vi "BIAS_Client_2.vi"() -> ()   [LabVIEW 2012]
uses:
  <userlib>/BIAS2/subvis/ROI_rect.ctl
  <userlib>/BIAS2/subvis/Imaging_State.ctl
  <userlib>/BIAS2/subvis/Frame_Controls.ctl
  <userlib>/BIAS2/subvis/ui/CameraParameters.ctl
  <vilib>/Utility/error.llb/DialogType.ctl
  <userlib>/BIAS2/subvis/zlock/ZLock.lvclass
  <userlib>/BIAS2/classes/CameraBase/CameraBase.lvclass
  <userlib>/BIAS2/subvis/ExposureSettings.ctl
  <vilib>/addons/h5labview2/file/H5Fmode.ctl
  <vilib>/event_ctls.llb/lveventtype.ctl
  <vilib>/addons/h5labview2/base/lib_path.vi
  <vilib>/addons/h5labview2/base/H5Equery.vi
  <vilib>/Utility/file.llb/Read From Spreadsheet File (DBL).vi
  <vilib>/addons/h5labview2/attrib/H5Aread.llb/H5Aread.xnode
  <vilib>/addons/h5labview2/dataset/H5Dread.llb/H5Dread.xnode
  <vilib>/addons/h5labview2/attrib/H5Awrite.llb/H5Awrite.xnode
  <vilib>/Analysis/NI_AALPro.lvlib
  <vilib>/addons/h5labview2/file/H5F.lvlib
  <vilib>/addons/h5labview2/group/H5G.lvlib
  <vilib>/addons/h5labview2/attrib/H5A.lvlib
panel:
  in  "files":T1 caption="Files"
  in  "stop":bool
  in  "tools_zoom":T2 caption="Zoom tools"
  in  "tools_view":cluster{"sel":bool, "in":bool, "out":bool} caption="View tools"
  in  "capture":T3 caption="Capture"
  out "stop_time":dbl=11.582550000000003
  out "busy":bool caption="Busy"
  out "recent_error":bool caption="Error"
  out "remote":bool caption="Remote"
  out "acquiring":bool caption="Acquiring"
  out "img_OD":T4(plugin-control)
  out "image_raw":sgl[][](array[numeric])
  in  "tabs":T5(tab)
  in  "binning":cluster{"x":u8, "y":u8}={"x"=1, "y"=1}
  in  "effective_pixel":dbl=5.9e-06 caption="effective pixel size"
  in  "rotation":u16(ring) items=["Do not rotate", "Rotate 90°", "Rotate 180°", "Rotate -90°"]
  out "cam_params":cluster{"String":string, "value":variant}[](array[cluster])=[{"String"="StatusInformation::LostBufferCount", "value"=variant(i64 0)}, {"String"="StatusInformation::LastBufferNumber", "value"=variant(u32 0)}, {"String"="StatusInformation::LastBufferCount", "value"=variant(i64 1)}, {"String"="StatusInformation::AcqInProgress", "value"=variant(bool FALSE)}, {"String"="CameraInformation::VendorName", "value"=variant(string "Point Grey Research")}, {"String"="CameraInformation::SerialNumberLow", "value"=variant(u32 11272219)}, {"String"="CameraInformation::SerialNumberHigh", "value"=variant(u32 11574529)}, {"String"="CameraInformation::ModelName", "value"=variant(string "Flea3 FL3-FW-03S1M")}, {"String"="CameraInformation::BusType", "value"=variant(string "FireWire")}, {"String"="CameraInformation::BaseAddress", "value"=variant(u32 4042260480)}, {"String"="CameraAttributes::TriggerDelay::Value", "value"=variant(dbl 0.0)}, {"String"="CameraAttributes::TriggerDelay::Mode", "value"=variant(string "Off")}, {"String"="CameraAttributes::Trigger::TriggerSource", "value"=variant(string "Source 0")}, {"String"="CameraAttributes::Trigger::TriggerParameter", "value"=variant(u32 0)}, {"String"="CameraAttributes::Trigger::TriggerMode", "value"=variant(string "Mode 1")}, {"String"="CameraAttributes::Trigger::TriggerActivation", "value"=variant(string "Level Low")}, {"String"="CameraAttributes::Trigger::SoftwareTrigger", "value"=variant(string "")}, {"String"="CameraAttributes::Temperature::Target", "value"=variant(dbl 2931.0)}, {"String"="CameraAttributes::Temperature::Mode", "value"=variant(string "UnknownEnumValue")}, {"String"="CameraAttributes::Temperature::Current", "value"=variant(dbl 3069.0)}, {"String"="CameraAttributes::Shutter::Value", "value"=variant(dbl 0.009999999776482582)}, {"String"="CameraAttributes::Shutter::Mode", "value"=variant(string "Absolute")}, {"String"="CameraAttributes::Sharpness::Value", "value"=variant(dbl 968.0)}, {"String"="CameraAttributes::Sharpness::Mode", "value"=variant(string "Off")}, {"String"="CameraAttributes::Gamma::Value", "value"=variant(dbl 1280.0)}, {"String"="CameraAttributes::Gamma::Mode", "value"=variant(string "Off")}, {"String"="CameraAttributes::Gain::Value", "value"=variant(dbl 10.0)}, {"String"="CameraAttributes::Gain::Mode", "value"=variant(string "Absolute")}, {"String"="CameraAttributes::FrameRate::Value", "value"=variant(dbl 480.0)}, {"String"="CameraAttributes::FrameRate::Mode", "value"=variant(string "Auto")}, {"String"="CameraAttributes::Brightness::Value", "value"=variant(dbl 0.0)}, {"String"="CameraAttributes::Brightness::Mode", "value"=variant(string "Absolute")}, {"String"="CameraAttributes::AutoExposure::Value", "value"=variant(dbl 6.0)}, {"String"="CameraAttributes::AutoExposure::Mode", "value"=variant(string "Off")}, {"String"="AcquisitionAttributes::Width", "value"=variant(u32 648)}, {"String"="AcquisitionAttributes::VideoMode", "value"=variant(string "Format 7, Mode 0, 648 x 488")}, {"String"="AcquisitionAttributes::Timeout", "value"=variant(u32 2000)}, {"String"="AcquisitionAttributes::SwapPixelBytes", "value"=variant(bool FALSE)}, {"String"="AcquisitionAttributes::Speed", "value"=variant(string "400 Mbps")}, {"String"="AcquisitionAttributes::ShiftPixelBits", "value"=variant(bool TRUE)}, {"String"="AcquisitionAttributes::ReserveDualPackets", "value"=variant(bool TRUE)}, {"String"="AcquisitionAttributes::ReceiveTimestampMode", "value"=variant(string "None")}, {"String"="AcquisitionAttributes::PixelSignedness", "value"=variant(string "Unsigned")}, {"String"="AcquisitionAttributes::PixelFormat", "value"=variant(string "Mono 16")}, {"String"="AcquisitionAttributes::PayloadSize", "value"=variant(u32 614400)}, {"String"="AcquisitionAttributes::PacketSize", "value"=variant(u32 3948)}, {"String"="AcquisitionAttributes::OverwriteMode", "value"=variant(string "Get Newest")}, {"String"="AcquisitionAttributes::OutputImageType", "value"=variant(string "Auto")}, {"String"="AcquisitionAttributes::OffsetY", "value"=variant(u32 0)}, {"String"="AcquisitionAttributes::OffsetX", "value"=variant(u32 0)}, {"String"="AcquisitionAttributes::IgnoreFirstFrame", "value"=variant(bool FALSE)}, {"String"="AcquisitionAttributes::Height", "value"=variant(u32 488)}, {"String"="AcquisitionAttributes::FrameInterval", "value"=variant(u32 19)}, {"String"="AcquisitionAttributes::Controller::StreamChannelMode", "value"=variant(string "Automatic")}, {"String"="AcquisitionAttributes::Controller::DesiredStreamChannel", "value"=variant(u32 0)}, {"String"="AcquisitionAttributes::BitsPerPixel", "value"=variant(string "12-bit")}, {"String"="AcquisitionAttributes::Bayer::Pattern", "value"=variant(string "Use hardware value")}, {"String"="AcquisitionAttributes::Bayer::GainR", "value"=variant(dbl 1.0)}, {"String"="AcquisitionAttributes::Bayer::GainG", "value"=variant(dbl 1.0)}, {"String"="AcquisitionAttributes::Bayer::GainB", "value"=variant(dbl 1.0)}, {"String"="AcquisitionAttributes::Bayer::Algorithm", "value"=variant(string "Bilinear")}] caption="Camera Parameters"
  in  "rois":T7(array[cluster])=[{"get"=FALSE, "set"=FALSE, "rect"={"left"=0, "top"=0, "right"=0, "bottom"=0}, "color"=16777224}, {"get"=FALSE, "set"=FALSE, "rect"={"left"=0, "top"=0, "right"=0, "bottom"=0}, "color"=6618880}, {"get"=FALSE, "set"=FALSE, "rect"={"left"=0, "top"=0, "right"=0, "bottom"=0}, "color"=16776960}, {"get"=FALSE, "set"=FALSE, "rect"={"left"=0, "top"=0, "right"=0, "bottom"=0}, "color"=4849919}]
  in  "camera name":string="XY_1_Flea3"
  out "camera model":string="Flea3 FL3-FW-03S1M, serial 0xB09D0100AC001B"
  in  "exposure":sgl=100.0 caption="exposure (ms)"
  out "location":string caption="camera location"
  out "roi_sensor":T6={"left"=0, "top"=0, "right"=640, "bottom"=480} caption="camera size"
  out "roi_capture":T6={"left"=0, "top"=0, "right"=640, "bottom"=480}
  out "keep":u8
  out "working dir":path
  out "current file":string
  in  "raw_ctrls":T8={"col_scheme"=0, "val_min"=100.0, "val_max"=16384.0, "automax"=FALSE} {"col_scheme" items=["Grayscale", "Rainbow", "Temperature", "-", "AlpineColors", "Amherst", "Aquamarine", "ArmyColors", "AtlanticColors", "AuroraColors", "AvocadoColors", "BeachColors", "BlueGreenYellow", "BrassTones", "BrightBands", "BrownCyanTones", "CandyColors", "CherryTones", "CMYKColors", "CoffeeTones", "DarkBands", "DarkRainbow", "DarkTerrain", "DeepSeaColors", "Default", "FallColors", "FruitPunchColors", "FuchsiaTones", "GrayTones", "GrayYellowTones", "GreenBrownTerrain", "GreenPinkTones", "IslandColors", "LabVIEW", "LakeColors", "LightTemperatureMap", "LightTerrain", "MintColors", "NeonColors", "NIST", "Pastel", "PearlColors", "PigeonTones", "PlumColors", "Rainbow", "RedBlueTones", "RedGreenSplit", "RoseColors", "RustTones", "SandyTerrain", "SiennaTones", "SolarColors", "SouthwestColors", "StarryNightColors", "SunsetColors", "TemperatureMap", "ThermometerColors", "ValentineTones", "WatermelonColors"]; "val_max" format="%_4g"; "val_min" format="%_4g"}
  in  "raw_list":i32(listbox)=-1 caption="Raw Frames"
  in  "hold_frames":bool caption="Hold last flat/dark frames"
  in  "histograms":bool caption="histogram"
  out "recent":string[](array[string])=["[31/10/14-12:50:53] Instance started, XY_1_Flea3"] caption="recent log messages"
  out "state":T9=enum."Quit" caption="system state"
  in  "last error":T10={"status"=FALSE, "code"=42, "description"="", "time"=timestamp(3029490000.67111 s since 1904-01-01)} caption="most recent error:" {"time" format="%<%H:%M:%S %d/%m/%y>T"}
  out "sequencer":T11(array[cluster])
  out "roi_current":T6
  out "image_data":u16[][][](array[numeric])
  out "frame":i32=-1 caption="display_frame"
  out "BLACS port":u16=1024
  out "image_size":i32[](array[numeric])
  out "attribs":variant[](array[variant])=[variant(i32 864), variant(i32 519), variant(i32 1176), variant(i32 878), variant(i64 0), variant(string "Freerun"), variant(u32 1), variant(u32 1), variant(i64 864), variant(i64 519), variant(i64 312), variant(i64 359), variant(dbl 100000.00149011612)]
  in  "Parameters":T12={"name"="XY_1_Flea3", "sdk"="IMAQdx_Flea3_Firewire", "serial"=49712223532875803, "port"=1024, "h5"=path "Y:/Experiments/rb_chip/connectiontable.h5", "zlock server"="localhost", "zlock port"=7339} {"serial" format="%x"}
  out "raw histograms":T13(array[cluster])
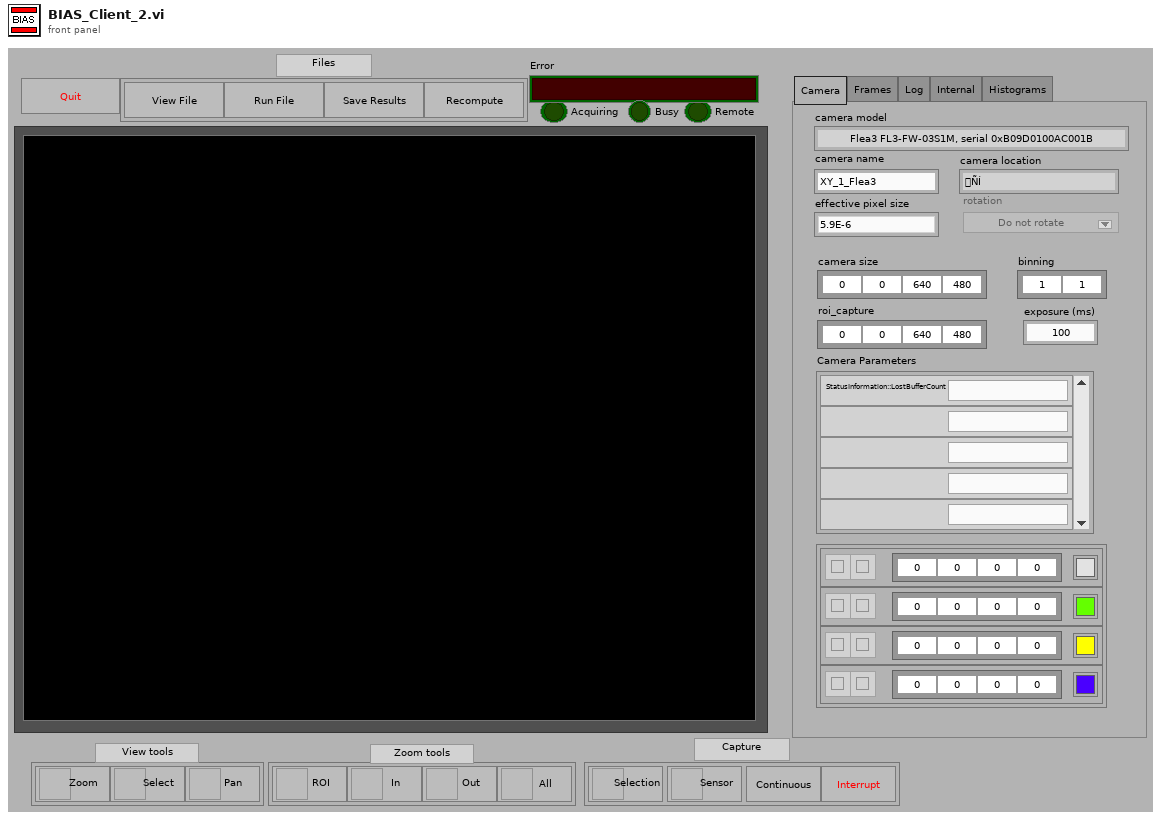
[diagram p1: front panel]
types:
  T1 = cluster{"open_file 2":bool, "open_file":bool, "save_file":bool, "open_file 3":bool}
  T2 = cluster{"sel":bool, "in":bool, "out":bool, "all":bool}
  T3 = cluster{"roi":bool, "chip":bool, "continuous":bool, "abort":bool}
  T4 = typedef "IMAQ Image.ctl" = refnum<image>
  T5 = enum32{"Camera", "Frames", "Log", "Internal", "Histograms"}
  T6 = typedef "ROI_rect.ctl" = cluster{"left":i32, "top":i32, "right":i32, "bottom":i32}
  T7 = cluster{"get":bool, "set":bool, "rect":T6, "color":u32}[]
  T8 = typedef "Frame_Controls.ctl" = cluster{"col_scheme":u16, "val_min":sgl, "val_max":sgl, "automax":bool}
  T9 = typedef "Imaging_State.ctl" = enum16{"<NULL>", "Init", "Read File", "Save File", "Idle", "Compute", "Redraw", "Draw Overlays", "Software trigger", "Acquire", "Fit", "Clear", "Quit"}
  T10 = cluster{"status":bool, "code":i32, "description":string, "time":timestamp}
  T11 = cluster{"name":string, "shots":string[], "ids":i32[]}[]
  T12 = typedef "CameraParameters.ctl" = cluster{"name":string, "sdk":string, "serial":u64, "port":u16, "h5":path, "zlock server":string, "zlock port":u32}
  T13 = cluster{"XY Graph":cluster{"X Values":dbl[], "Histogram: h(x)":i32[]}}[]
  T14 = typedef "DialogType.ctl" = u16
  T15 = typedef "ExposureSettings.ctl" = cluster{"exposure":dbl, "external":bool, "roi":T6, "frames":i32, "binning":cluster{"x":u8, "y":u8}}
  T16 = typedef "H5F.lvlib/H5Fmode.ctl" = enum16{"read-only", "read-write", "overwrite", "create new", "open or create"}
  T17 = typedef "Image Type" = u32
  T18 = cluster{"sensor_width":u16, "sensor_width":u16, "sensor_width":u16, "sensor_height":u16}
  T19 = cluster{"X Values":dbl[], "Histogram: h(x)":i32[]}
  T20 = cluster{"Histogram Graph":cluster{"X Values":dbl[], "Histogram: h(x)":i32[]}}
  T21 = typedef "hid_t.ctl" = i32
  T22 = cluster{"name":string, "shots":string[], i32[]}[]
  T23 = typedef "lveventtype.ctl" = enum32{"Null", "Timeout", "Annotation Menu Selection", "Annotation Menu Selection?", "App Instance Close", "App Instance Close?", "Autoscale Range Change", "Cell Edit", "Cell Edit?", "Cursor Grab", "Cursor Grab?", "Cursor Menu Selection", "Cursor Menu Selection?", "Cursor Move", "Cursor Release", "Data Change", "Direction Change", "Display State Change", "Drag Ended", "Drag Enter", "Drag Leave", "Drag Over", "Drag Source Update", "Drag Starting", "Drag Starting?", "Drop", "Exec State Change", "Key Down", "Key Down?", "Key Repeat", "Key Repeat?", "Key Up", "Listbox Double Click", "Menu Activation?", "Menu Selection (App)", "Menu Selection? (App)", "Menu Selection (User)", "Mouse Down", "Mouse Down?", "Mouse Enter", "Mouse Leave", "Mouse Move", "Mouse Up", "NI Security User Change (App)", "Pane Size", "Panel Close", "Panel Close?", "Panel Resize", "Plot Attribute Change", "Scale Range Change", "Shortcut Menu Activation?", "Shortcut Menu Selection (App)", "Shortcut Menu Selection? (App)", "Shortcut Menu Selection (User)", "Tree Double Click", "Tree Drag", "Tree Drag?", "Tree Drop", "Tree Drop?", "Tree Item Close", "Tree Item Close?", "Tree Item Open", "Tree Item Open?", "Value Change"}
  T24 = cluster{"Global Rectangle":i32[], "Contours":cluster{"Contour Type":u32, "ROI Type":u32, "Points":i32[]}[]}
  T25 = typedef "ROI Descriptor" = cluster{"Global Rectangle":i32[], "Contours":cluster{"ID":enum32{"External", "Internal"}, "Type":u32, "Coordinates":i32[]}[]}
  T26 = cluster{"Contour Type":u32, "ROI Type":u32, "Points":i32[]}[]
  T27 = cluster{"FinalVal[0]":bool, "FinalVal[1]":bool, "FinalVal[2]":bool}
  T28 = cluster{"all rows[0]":dbl, "all rows[1]":dbl, "all rows[2]":dbl}
  T29 = cluster{"get":bool, "set":bool, "rect":T6, "color":u32}
  T30 = cluster{"Value":u8, "Value":u8, "Value":u8, "Value":u8}
  T31 = cluster{"col_scheme":u16, "val_min":sgl, "val_max":sgl, "automax":bool}
  T32 = enum16{"Standard", "Buffered", "CRLF", "Immediate"}
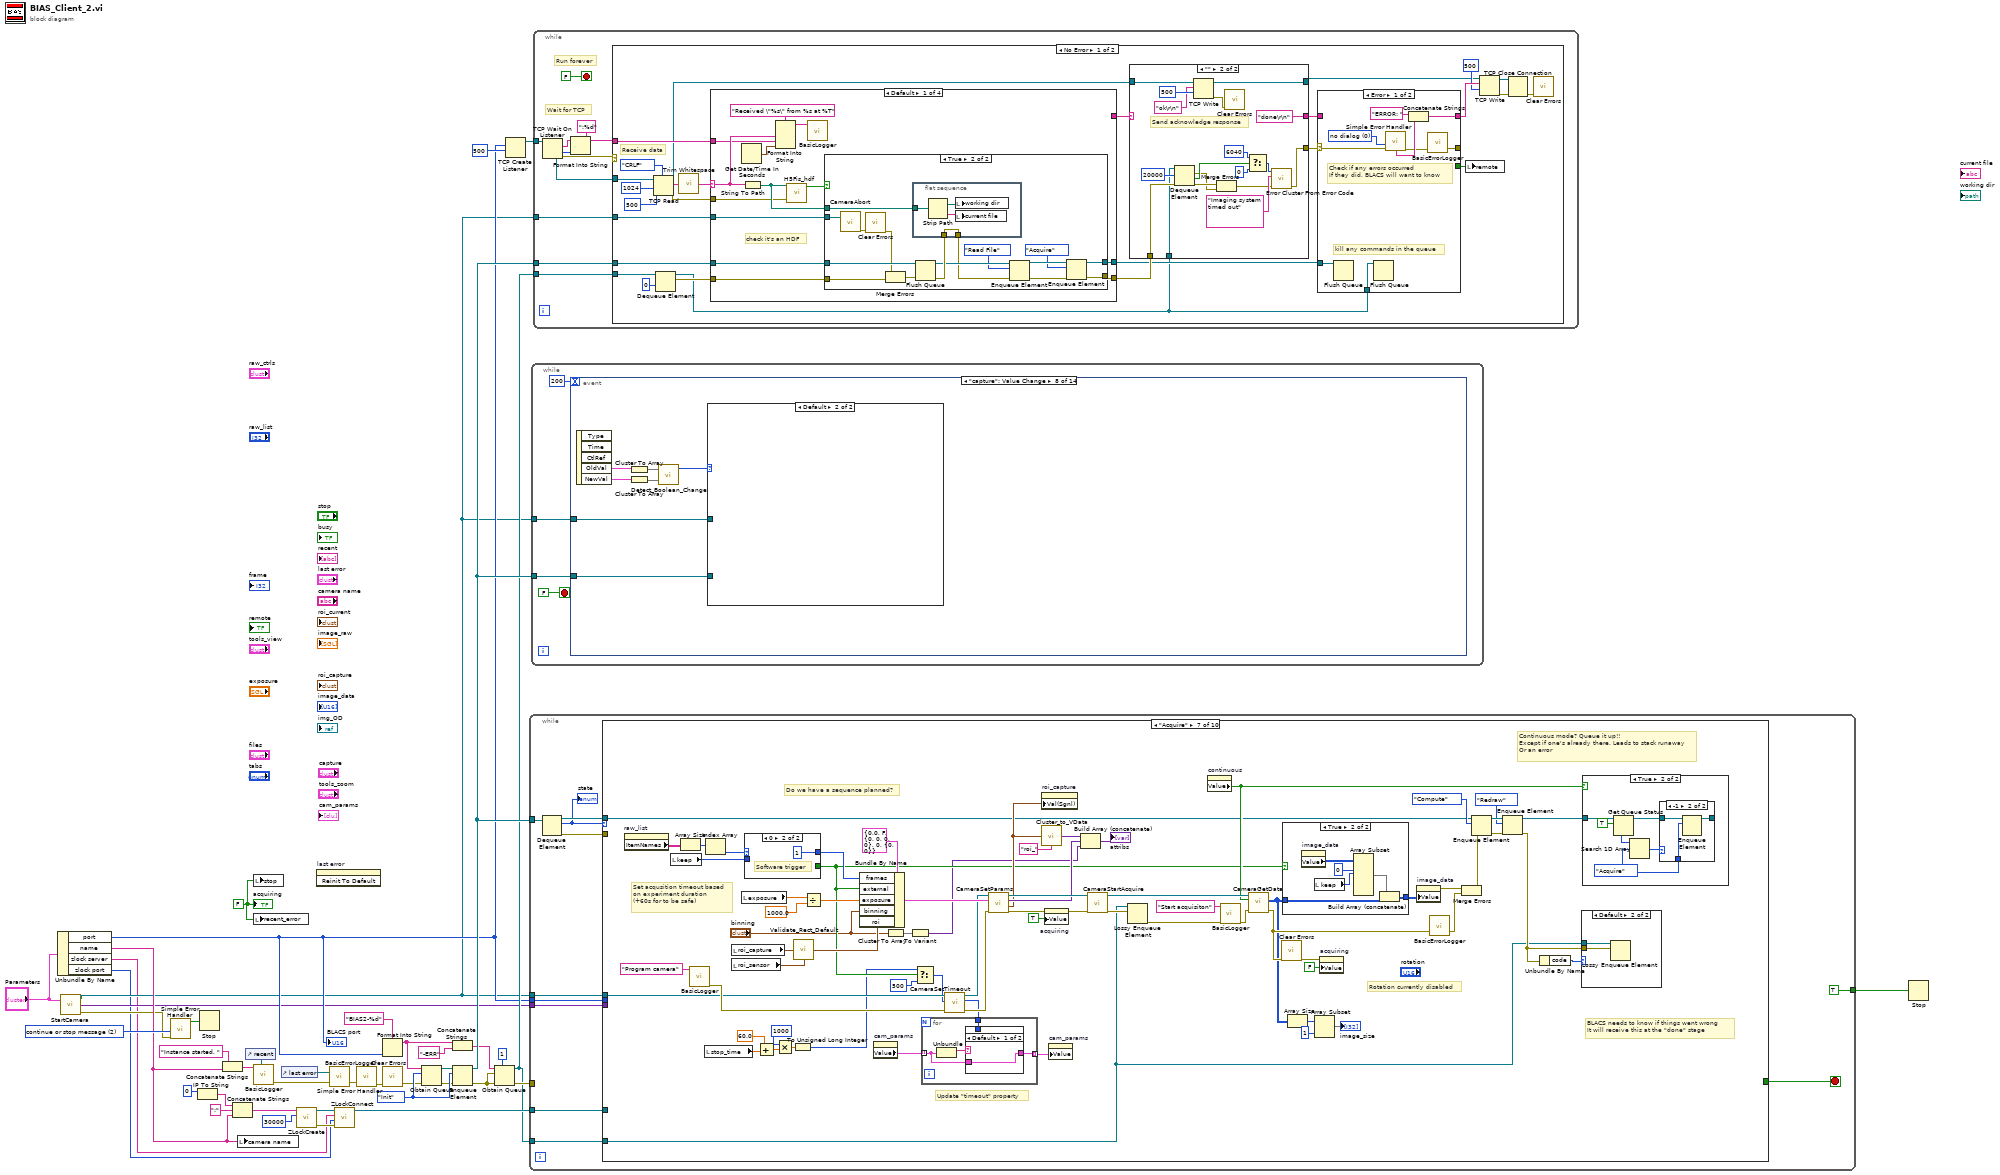
[diagram p0: block diagram]
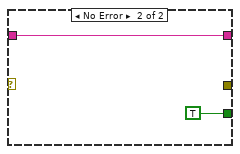
[diagram p2: hidden frame]
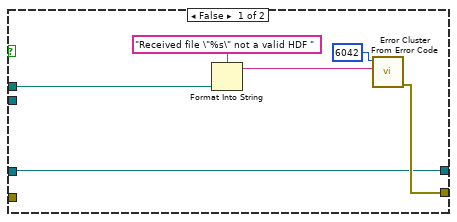
[diagram p4: hidden frame]
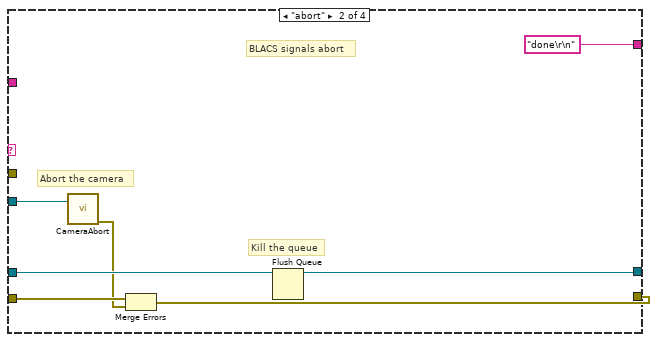
[diagram p5: hidden frame]
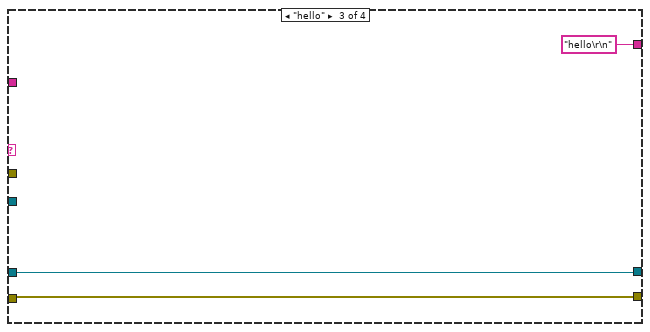
[diagram p6: hidden frame]
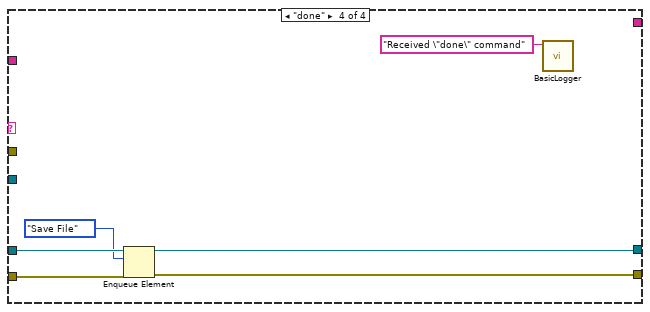
[diagram p7: hidden frame]
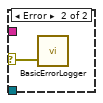
[diagram p8: hidden frame]
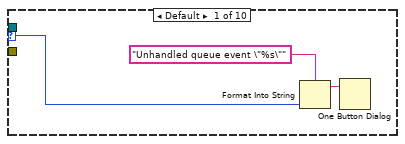
[diagram p9: hidden frame]
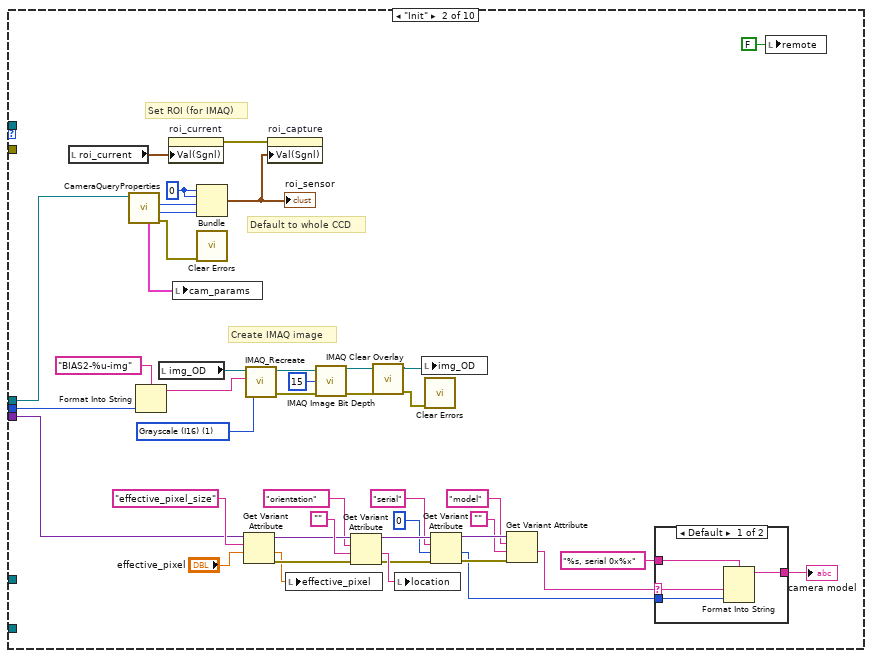
[diagram p10: hidden frame]
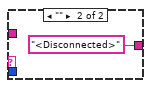
[diagram p11: hidden frame]
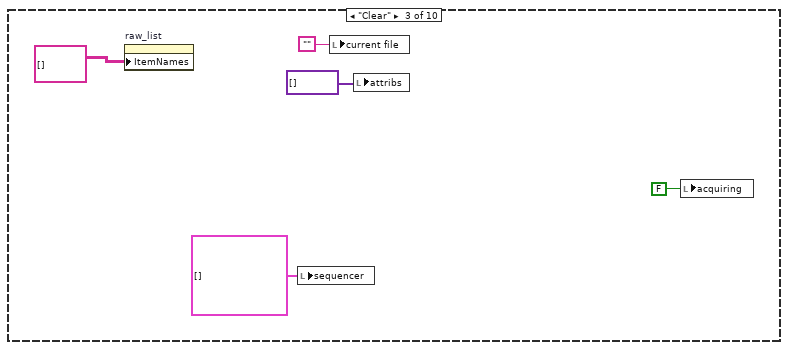
[diagram p12: hidden frame]
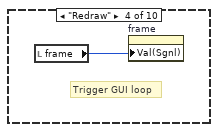
[diagram p13: hidden frame]
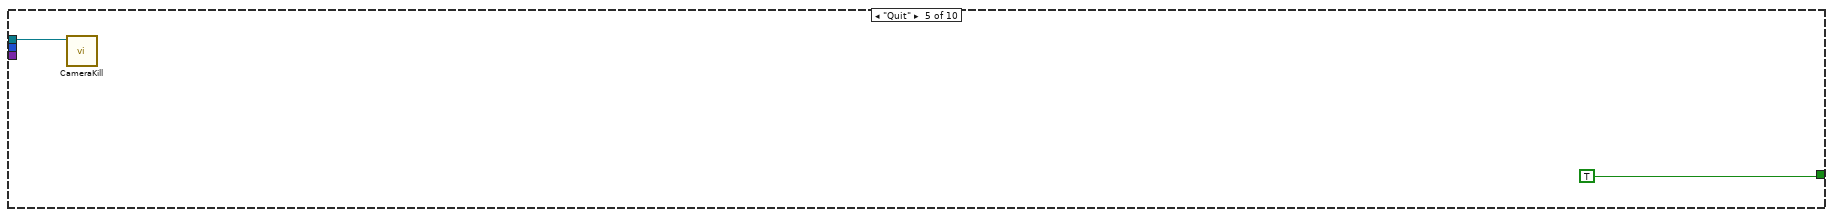
[diagram p14: hidden frame]
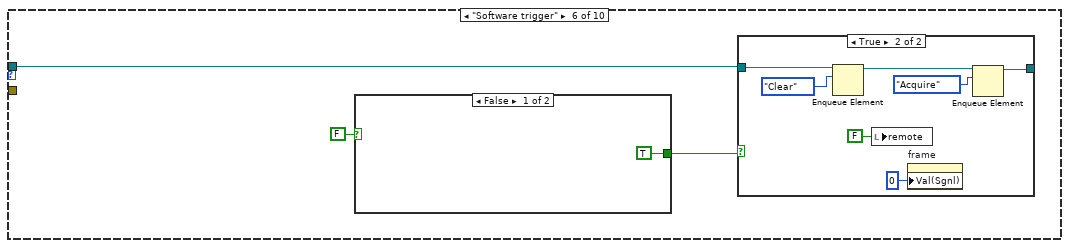
[diagram p15: hidden frame]
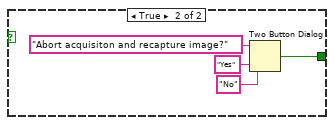
[diagram p17: hidden frame]
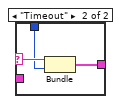
[diagram p19: hidden frame]
diagram:
  w24 = T14 2 items=["no dialog", "OK message", "continue or stop message", "OK message + warnings", "continue/stop + warnings"] ("type of dialog (OK msg:1)")
  w27 = FALSE ("acquiring")
  w41 = Imaging_State."Init" ("Imaging_State")
  n1 = Unbundle By Name("Parameters") -> ("port"=w7:u16, "name"=w8:string, "zlock server"=w3:string, "zlock port"=w2:u32)
  "BLACS port" <- w7
  n2 = call <userlib>:"StartCamera.vi"("Parameters"="Parameters") -> ("camera"=w6:refnum<class "CameraBase.lvclass">, "params"=w5:variant, "error out"=w4:errorcluster)  [unwired: 1 in]
  n3 = call <vilib>:"Simple Error Handler.vi"("type of dialog (OK msg:1)"=w24, "error in (no error)"=w4) -> ("error?"=w25:bool)  [unwired: 3 in, 4 out]
  n4 = IP To String(2:u32 0 ("net address")) -> (0:w19:string)  [unwired: 1 in]
  n5 = Stop(stop? (T)=w25) -> ()
  n6 = Concatenate Strings("Instance started, " ("string"), w8) -> (w28:string)
  n7 = Concatenate Strings(w19, ":" ("string"), w8) -> (w20:string)
  n8 = local write "camera name"(w8) -> ()
  n9 = control-ref of="recent"() -> (w30:refnum<vi>)
  n10 = local write "stop"(w27) -> ()
  n11 = local write "recent_error"(w27) -> ()
  n12 = call <userlib>:"BasicLogger.vi"("indicator"=w30, "text"=w28) -> ("error out"=w31:errorcluster)  [unwired: 5 in, 1 out]
  n13 = control-ref of="last error"() -> (w35:refnum<vi>)
  n14 = call <userlib>:"ZLockCreate.vi"("timeout (500ms)"=30000, "app name"=w20) -> ("error out"=w22:errorcluster, "ZLock out"=w23:refnum<class "ZLock.lvclass">)  [unwired: 4 in]
  n15 = invoke on="last error" class="Clust (strict)" method="Reinit To Default"() -> ()  [unwired: 3 in, 3 out]
  n16 = call <userlib>:"BasicErrorLogger.vi"("error in"=w31, "indicator"=w35) -> ("error out"=w34:errorcluster)  [unwired: 1 out]
  n17 = call-dynamic "ZLockConnect.vi"("error in (no error)"=w22, "port (7339)"=w2, "host"=w3, "ZLock in"=w23) -> ("ZLock out"=w21:refnum<class "ZLock.lvclass">)  [unwired: 6 in, 1 out]
  n18 = call <vilib>:"Simple Error Handler.vi"("error in (no error)"=w34) -> ("error out"=w33:errorcluster)  [unwired: 4 in, 4 out]
  n19 = Format Into String(format string="BIAS2-%d" ("name (unnamed)"), w7) -> (resulting string=w15:string)  [unwired: 2 in, 1 out]
  n20 = call <vilib>:"Clear Errors.vi"("error in (no error)"=w33) -> ("error out"=w32:errorcluster)  [unwired: 6 in]
  n21 = Obtain Queue(name (unnamed)=w15, element data type=w41, error in (no error)=w32) -> (queue out=w42:refnum<queue>, error out=w40:errorcluster)  [unwired: 2 in, 1 out]
  n22 = Concatenate Strings(w15, "-ERR" ("name (unnamed)")) -> (w13:string)
  n23 = Enqueue Element(queue=w42, element=w41, error in (no error)=w40) -> (queue out=w37:refnum<queue>, error out=w12:errorcluster)  [unwired: 1 in, 1 out]
  n24 = Obtain Queue(max queue size (-1, unlimited)=1, name (unnamed)=w13, element data type=w12, error in (no error)=w12) -> (queue out=w9:refnum<queue>, error out=w16:errorcluster)  [unwired: 1 in, 1 out]
  n25 = TCP Create Listener(9:500 ("timeout ms (25000)"), 10:w7) -> (3:w36:refnum<k5>)  [unwired: 3 in, 2 out]
  n26 = while {
    tunnel: [TRUE] -> w39
    tunnel: w6 -> [w49]
    tunnel: w37 -> [w45]
    tunnel: w21 -> [w48]
    tunnel: w7 -> [w47]
    tunnel: w5 -> [w44]
    tunnel: w16 -> [_]
    tunnel: w9 -> [w43]
    stop <- w50 stop-if-true
    n27 = Dequeue Element(queue=w45) -> (queue out=w53:refnum<queue>, element=w46:T9, error out=w52:errorcluster)  [unwired: 2 in, 1 out]
    "state" <- w46
    n28 = case shown="\"Acquire\"" w46 {
      selector: w46 -> [w55 _ _ _ _ _ _ _ _ _]
      tunnel: w53 -> [_ _ _ _ _ w114 w133 _ w247 w467]
      tunnel: w52 -> [_ _ _ _ _ _ _ _ _ _]
      tunnel: [_ _ _ _ TRUE _ _ _ _ _] -> w50
      tunnel: w49 -> [_ w83 _ _ w111 _ w167 _ _ _]
      tunnel: w48 -> [_ _ _ _ _ _ _ _ w242 w468]
      tunnel: w47 -> [_ w78 _ _ _ _ _ _ _ _]
      tunnel: w44 -> [_ w62 _ _ _ _ _ _ _ _]
      tunnel: w43 -> [_ _ _ _ _ _ w129 _ w241 w466]
      frame Default {
        n29 = Format Into String(format string="Unhandled queue event \"%s\"", w55) -> (resulting string=w54:string)  [unwired: 2 in, 1 out]
        n30 = One Button Dialog(message=w54) -> ()  [unwired: 1 in, 1 out]
      }
      frame "Init" {
        w82 = u16 0 ("sensor_width")
        w98 = T17 1 items=["Grayscale (U8)", "Grayscale (I16)", "Grayscale (SGL)", "Complex (CSG)", "RGB (U32)", "HSL (U32)", "RGB (U64)", "Grayscale (U16)"] ("type")
        # "Create IMAQ image"
        # "Default to whole CCD"
        # "Set ROI (for IMAQ)"
        n31 = local read "roi_current"() -> (w93:T6)
        n32 = call-dynamic "CameraQueryProperties.vi"("CameraBase in"=w83) -> ("error out"=w84:errorcluster, "sensor_height"=w92:u16, "sensor_width"=w91:u16, "cam_params"=w90:cluster{"String":string, "value":variant}[])  [unwired: 6 in, 1 out]
        n33 = Format Into String(format string="BIAS2-%u-img", w78) -> (resulting string=w79:string)  [unwired: 2 in, 1 out]
        n34 = local read "img_OD"() -> (w99:T4)
        n35 = property on="roi_current" class="Clust (strict)"("Val(Sgnl)"=w93) -> (error out=w94:errorcluster)  [unwired: 2 in, 1 out]
        n36 = local write "cam_params"(w90) -> ()
        n37 = Bundle("sensor_width"=w82, "sensor_width"=w82, "sensor_width"=w91, "sensor_height"=w92) -> (w81:T18)  [unwired: 1 in]
        "roi_sensor" <- w81
        n38 = call <vilib>:"Clear Errors.vi"("error in (no error)"=w84) -> ()  [unwired: 6 in, 1 out]
        n39 = Get Variant Attribute(Variant=w62, name="effective_pixel_size", default value (empty Variant)="effective_pixel") -> (duplicate Variant=w71:variant, value=w64:dbl, error out=w74:errorcluster)  [unwired: 1 in, 1 out]
        n40 = call <userlib>:"IMAQ_Recreate.vi"("type"=w98, "name"=w79, "image in"=w99) -> ("error out"=w95:errorcluster, "image out"=w97:T4)  [unwired: 3 in]
        n41 = property on="roi_capture" class="Clust (strict)"(error in=w94, "Val(Sgnl)"=w81) -> ()  [unwired: 1 in, 2 out]
        n42 = local write "effective_pixel"(w64) -> ()
        n43 = call "IMAQ Image Bit Depth"("Image"=w97, "Bit Depth (0)"=u32 15, "error in (no error)"=w95) -> ("Image Out"=w88:T4, "error out"=w89:errorcluster)  [unwired: 10 in, 1 out]
        n44 = Get Variant Attribute(Variant=w71, name="orientation", default value (empty Variant)="", error in=w74) -> (duplicate Variant=w72:variant, value=w76:string, error out=w75:errorcluster)  [unwired: 1 out]
        n45 = call "IMAQ Clear Overlay"("error in (no error)"=w89, "Image"=w88) -> ("error out"=w86:errorcluster, "Image Out"=w87:T4)  [unwired: 8 in]
        n46 = local write "location"(w76) -> ()
        n47 = local write "img_OD"(w87) -> ()
        n48 = call <vilib>:"Clear Errors.vi"("error in (no error)"=w86) -> ()  [unwired: 6 in, 1 out]
        n49 = Get Variant Attribute(Variant=w72, name="serial", default value (empty Variant)=u64 0, error in=w75) -> (duplicate Variant=w69:variant, value=w67:u64, error out=w70:errorcluster)  [unwired: 1 out]
        n50 = Get Variant Attribute(Variant=w69, name="model", default value (empty Variant)="", error in=w70) -> (value=w68:string)  [unwired: 3 out]
        n51 = case shown="Default" w68 {
          selector: w68 -> [w101 _]
          tunnel: [w103 "<Disconnected>"] -> w58
          tunnel: w67 -> [w102 _]
          tunnel: "%s, serial 0x%x" ("format string") -> [w100 _]
          frame Default {
            n52 = Format Into String(format string=w100, w101, w102) -> (resulting string=w103:string)  [unwired: 2 in, 1 out]
          }
          frame "" {
          }
        }
        "camera model" <- w58
        n53 = local write "remote"(FALSE ("remote")) -> ()
      }
      frame "Clear" {
        n54 = property on="raw_list" class="MCListbox (strict)"("ItemNames"=string[][] [] ("sequence")) -> ()  [unwired: 2 in, 2 out]
        n55 = local write "sequencer"(T11 [] ("sequencer")) -> ()
        n56 = local write "current file"("") -> ()
        n57 = local write "attribs"(variant[] []) -> ()
        n58 = local write "acquiring"(FALSE ("pending")) -> ()
      }
      frame "Redraw" {
        # "Trigger GUI loop"
        n59 = local read "frame"() -> (w110:i32)
        n60 = property on="frame" class="DigNum (strict)"("Val(Sgnl)"=w110) -> ()  [unwired: 2 in, 2 out]
      }
      frame "Quit" {
        n61 = call-dynamic "CameraKill.vi"("CameraBase in"=w111) -> ()  [unwired: 9 in, 2 out]
      }
      frame "Software trigger" {
        n62 = case shown="False" FALSE {
          tunnel: [TRUE ("T button?") w125] -> w115
          frame False {
          }
          frame True {
            n63 = Two Button Dialog(message="Abort acquisiton and recapture image?", 1:"No" ("F button name (\"Cancel\")"), 2:"Yes" ("T button name (\"OK\")")) -> (T button?=w125:bool)
          }
        }
        n64 = case shown="True" w115 {
          tunnel: [w116 w122] -> _
          tunnel: w114 -> [w116 w121]
          frame False {
          }
          frame True {
            n65 = Enqueue Element(queue=w121, element=Imaging_State."Clear") -> (queue out=w120:refnum<queue>)  [unwired: 2 in, 2 out]
            n66 = local write "remote"(FALSE ("remote")) -> ()
            n67 = property on="frame" class="DigNum (strict)"("Val(Sgnl)"=0 ("Value (Signaling)")) -> ()  [unwired: 2 in, 2 out]
            n68 = Enqueue Element(queue=w120, element=Imaging_State."Acquire") -> (queue out=w122:refnum<queue>)  [unwired: 2 in, 2 out]
          }
        }
      }
      frame "Acquire" {
        # "Update \"timeout\" property"
        # "Rotation currently disabled"
        # "Set acqusition timeout based\non experiment duration\n(+60s for to be safe)"
        # "BLACS needs to know if things went wrong\nIt will receive this at the \"done\" stage"
        # "Continuous mode? Queue it up!!\nExcept if one's already there. Leads to stack runaway\nOr an error"
        # "Do we have a sequence planned?"
        n69 = property on="raw_list" class="MCListbox (strict)"() -> ("ItemNames"=w178:string[][])  [unwired: 2 in, 2 out]
        n70 = local read "keep"() -> (w171:u8)
        n71 = Array Size(array=w178) -> (size(s)=w177:i32[])
        n72 = call <userlib>:"BasicLogger.vi"("text"="Program camera") -> ("error out"=w168:errorcluster)  [unwired: 6 in, 1 out]
        n73 = local read "stop_time"() -> (w162:dbl)
        n74 = Index Array(array=w177) -> (element=w176:i32)  [unwired: 1 in]
        n75 = local read "roi_capture"() -> (w192:T6)
        n76 = local read "roi_sensor"() -> (w187:T6)
        n77 = local read "exposure"() -> (w196:sgl)
        n78 = case shown="0" w176 {
          selector: w176 -> [w225 _]
          tunnel: [w226 1] -> w153
          tunnel: [TRUE ("external") _] -> w144
          tunnel: w171 -> [w224 _]
          frame Default {
            n79 = Subtract(x=w225, y=w224) -> (x-y=w226:i32)
          }
          frame 0 {
            # "Software trigger"
          }
        }
        n80 = Add(x=60.0, y=w162) -> (x+y=w163:dbl)
        n81 = Multiply(x=u32 1000 ("col"), y=w163) -> (x*y=w170:dbl)
        n82 = To Unsigned Long Integer(number=w170) -> (unsigned 32bit integer=w143:u32)
        n83 = call <userlib>:"Validate_Rect_Default.vi"("rect"=w192, "default"=w187) -> ("out"=w157:T6)
        n84 = Divide(x=w196, y=sgl 1000.0) -> (x/y=w191:sgl)
        n85 = Bundle By Name(cluster=T15 {"exposure"=0.0, "external"=FALSE, "roi"={"left"=0, "top"=0, "right"=0, "bottom"=0}, "frames"=0, "binning"={"x"=0, "y"=0}} ("settings"), "frames"=w153, "external"=w144, "exposure"=w191, "binning"="binning", "roi"=w157) -> (w190:T15)
        n86 = property on="cam_params" class="Arr (strict)"() -> ("Value"=w152:cluster{"String":string, "value":variant}[])  [unwired: 2 in, 2 out]
        n87 = Cluster To Array(cluster="binning") -> (array=w134:u8[])
        n88 = To Variant(anything=w134) -> (Variant=w135:variant)
        n89 = Select(t=w143, s=w144, f=u32 500) -> (s? t:f=w142:u32)
        n90 = call-dynamic "CameraSetTimeout.vi"("error in (no error)"=w168, "Timeout"=w142, "CameraBase in"=w167) -> ("error out"=w166:errorcluster, "Timeout set"=w164:u32, "CameraBase out"=w165:refnum<class "CameraBase.lvclass">)  [unwired: 6 in]
        n91 = for {
          tunnel: w152 -> [w204] mode=indexing
          tunnel: w164 -> [w205]
          tunnel: [w207] -> w151 mode=indexing
          n92 = Unbundle(w204) -> ("String"=w206:string)  [unwired: 1 out]
          n93 = case shown="Default" w206 {
            selector: w206 -> [_ w210]
            tunnel: [w208 w211] -> w207
            tunnel: w205 -> [_ w209]
            tunnel: w204 -> [w208 _]
            frame Default {
            }
            frame "Timeout" {
              n94 = Bundle(w210, "Timeout set"=w209) -> (w211:cluster{string, "Timeout set":u32})  [unwired: 1 in]
            }
          }
        }
        n95 = call-dynamic "CameraSetParams.vi"("error in (no error)"=w166, "settings"=w190, "CameraBase in"=w165) -> ("error out"=w183:errorcluster, "roi_out"=w159:T6, "attributes"=w175:variant[], "CameraBase out"=w182:refnum<class "CameraBase.lvclass">)  [unwired: 5 in]
        n96 = call <userlib>:"Cluster_to_VData.vi"("cluster"=w159, "prefix"="roi_") -> ("vdata"=w174:variant[])
        n97 = property on="roi_capture" class="Clust (strict)"("Val(Sgnl)"=w159) -> ()  [unwired: 2 in, 2 out]
        n98 = property on="acquiring" class="Bool (strict)"(error in=w183, "Value"=TRUE ("acquiring")) -> (error out=w180:errorcluster)  [unwired: 1 in, 1 out]
        n99 = property on="cam_params" class="Arr (strict)"("Value"=w151) -> ()  [unwired: 2 in, 2 out]
        n100 = Build Array (concatenate)(w174, w175, w135) -> (→"attribs":variant[])
        n101 = call-dynamic "CameraStartAcquire.vi"("error in (no error)"=w180, "CameraBase in"=w182) -> ("error out"=w131:errorcluster, "CameraBase out"=w181:refnum<class "CameraBase.lvclass">)  [unwired: 8 in]
        n102 = Lossy Enqueue Element(queue=w129, element=w131) -> (error out=w132:errorcluster)  [unwired: 1 in, 3 out]
        n103 = property on="continuous" class="Bool (strict)"() -> ("Value"=w156:bool)  [unwired: 2 in, 2 out]
        n104 = call <userlib>:"BasicLogger.vi"("error in"=w132, "text"="Start acquisiton") -> ("error out"=w179:errorcluster)  [unwired: 5 in, 1 out]
        n105 = call-dynamic "CameraGetData.vi"("error in (no error)"=w179, "keep open?"=w156, "CameraBase in"=w181) -> ("error out"=w194:errorcluster, "image_data"=w140:u16[][][])  [unwired: 6 in, 1 out]
        n106 = call <vilib>:"Clear Errors.vi"("error in (no error)"=w194) -> ("error out"=w184:errorcluster)  [unwired: 6 in]
        n107 = case shown="True" w144 {
          tunnel: [w197 w200] -> w160
          tunnel: w140 -> [w197 w198]
          frame False {
          }
          frame True {
            n108 = property on="image_data" class="Arr (strict)"() -> ("Value"=w199:u16[][][])  [unwired: 2 in, 2 out]
            n109 = local read "keep"() -> (w202:u8)
            n110 = Array Subset(array=w199, index (dim 0)=0 ("index"), length (dim 0)=w202) -> (w201:u16[][][])  [unwired: 4 in]
            n111 = Build Array (concatenate)(w201, w198) -> (w200:u16[][][])
          }
        }
        n112 = Array Size(array=w140) -> (size(s)=w139:i32[])
        n113 = Array Subset(array=w139, index=1) -> (→"image_size":i32[])  [unwired: 1 in]
        n114 = property on="acquiring" class="Bool (strict)"(error in=w184, "Value"=FALSE ("acquiring")) -> ()  [unwired: 1 in, 2 out]
        n115 = property on="image_data" class="Arr (strict)"("Value"=w160) -> (error out=w155:errorcluster)  [unwired: 2 in, 1 out]
        n116 = call <userlib>:"BasicErrorLogger.vi"("error in"=w194) -> ("error out"=w154:errorcluster)  [unwired: 1 in, 1 out]
        n117 = Merge Errors(w155, w154) -> (w147:errorcluster)
        n118 = Enqueue Element(queue=w133, element=Imaging_State."Compute", error in (no error)=w147) -> (queue out=w150:refnum<queue>, error out=w146:errorcluster)  [unwired: 1 in, 1 out]
        n119 = Enqueue Element(queue=w150, element=Imaging_State."Redraw", error in (no error)=w146) -> (queue out=w130:refnum<queue>, error out=w145:errorcluster)  [unwired: 1 in, 1 out]
        n120 = Unbundle By Name(w145) -> ("code"=w172:i32)
        n121 = case shown="Default" w172 {
          tunnel: w145 -> [_ w213]
          tunnel: w129 -> [_ w212]
          frame 0, 5024 {
            # "Fine or Abort"
          }
          frame Default {
            n122 = Lossy Enqueue Element(queue=w212, element=w213) -> ()  [unwired: 1 in, 4 out]
          }
        }
        n123 = case shown="True" w156 {
          tunnel: w130 -> [_ w219]
          frame False {
          }
          frame True {
            w214 = Imaging_State."Acquire" ("element")
            n124 = Get Queue Status(queue=w219, return elements? (F)=TRUE) -> (queue out=w215:refnum<queue>, elements=w217:T9[])  [unwired: 1 in, 6 out]
            n125 = Search 1D Array(1D array=w217, element=w214) -> (index of element=w216:i32)  [unwired: 1 in]
            n126 = case shown="-1" w216 {
              tunnel: [w220 w223] -> _
              tunnel: w215 -> [w220 w222]
              tunnel: w214 -> [_ w221]
              frame Default {
              }
              frame -1 {
                n127 = Enqueue Element(queue=w222, element=w221) -> (queue out=w223:refnum<queue>)  [unwired: 2 in, 2 out]
              }
            }
          }
        }
      }
      frame "Compute" {
        n128 = case shown="True" "histograms" {
          frame False {
          }
          frame True {
            # "Raw image histograms (very slow)"
            n129 = property on="image_data" class="Arr (strict)"() -> ("Value"=w230:u16[][][])  [unwired: 2 in, 2 out]
            n130 = for {
              tunnel: w230 -> [w238] mode=indexing
              tunnel: [w234] -> w231 mode=indexing
              n131 = Array Size(array=w238) -> (size(s)=w240:i32[])
              n132 = Multiply Array Elements(1:w240) -> (0:w239:i32)
              n133 = Reshape Array(w238, w239) -> (w237:u16[])
              n134 = call <vilib>:"General Histogram.vi"("X"=w237, "max"=16384.0, "min"=0.0, "# bins"=400 ("intervals")) -> ("Histogram Graph"=w235:T19)  [unwired: 7 in, 4 out]
              n135 = Bundle("Histogram Graph"=w235) -> (w234:T20)  [unwired: 1 in]
            }
            "raw histograms" <- w231
          }
        }
      }
      frame "Read File" {
        n136 = local write "recent_error"(FALSE ("recent_error")) -> ()
        n137 = local read "working dir"() -> (w246:path)
        n138 = local read "current file"() -> (w245:string)
        n139 = property on="continuous" class="Bool (strict)"("Value"=FALSE ("continuous")) -> ()  [unwired: 2 in, 2 out]
        n140 = case shown="Default" w245 {
          selector: w245 -> [w273 _]
          tunnel: w247 -> [w250 _]
          tunnel: w246 -> [w274 _]
          tunnel: w242 -> [w265 _]
          tunnel: w241 -> [w248 _]
          frame Default {
            n141 = local read "camera name"() -> (w276:string)
            n142 = Build Path(base path=w274, name or relative path=w273) -> (appended path=w260:path)
            n143 = Path To String(path=w260) -> (string=w266:string)
            n144 = call-dynamic "ZLockAcquire.vi"("key"=w266, "ZLock in"=w265) -> ("error out"=w259:errorcluster, "key out"=w263:string, "ZLock out"=w264:refnum<class "ZLock.lvclass">)  [unwired: 7 in]
            n145 = Concatenate Strings("Read file  " ("text"), w273) -> (w278:string)
            n146 = call <vilib>:"H5Fopen.vi"("error in (no error)"=w259, "mode (read-only)"=H5Fmode."read-only", "path"=w260) -> ("error out"=w255:errorcluster, "ref out"=w258:T21)  [unwired: 3 in]
            n147 = Concatenate Strings("/devices/" ("Name"), w276) -> (w254:string)
            n148 = call <userlib>:"BasicLogger.vi"("text"=w278) -> ()  [unwired: 6 in, 2 out]
            n149 = call <vilib>:"H5Gopen.vi"("error in (no error)"=w255, "name"=w254, "ref in"=w258) -> ("error out"=w256:errorcluster, "group out"=w257:T21)  [unwired: 4 in]
            n150 = case shown="Error" w256 {
              selector: w256 -> [_ w453]
              tunnel: [w337 w452] -> w253
              tunnel: w257 -> [w328 _]
              tunnel: [w312 w455] -> w252
              tunnel: [w331 w451] -> w272
              tunnel: [w334 w456] -> w271
              tunnel: w258 -> [w311 w455]
              frame No Error {
                w300 = string[] []
                w297 = "EXPOSURES" ("name")
                # "When is the experiment scheduled to finish?"
                n151 = xnode "H5Aread.xnode"("default"=0.0, "attrib name"="exposure_time" ("attribute"), "ref in"=w328) -> ("error out"=w322:errorcluster, "data"=w325:dbl, "ref out"=w324:i32)  [unwired: 3 in, 1 out]
                n152 = Multiply(x=w325, y=1000.0) -> (x*y=w338:dbl)
                n153 = local write "exposure"(w338) -> ()
                n154 = xnode "H5Aread.xnode"("error in (no error)"=w322, "default"="", "attrib name"="orientation" ("attribute"), "ref in"=w324) -> ("error out"=w306:errorcluster, "data"=w320:string, "ref out"=w305:i32)  [unwired: 2 in, 1 out]
                "location" <- w320
                n155 = Concatenate Strings("/images/" ("Name"), w320) -> (w318:string)
                n156 = xnode "H5Aread.xnode"("object name"="/devices/pulseblaster_0" ("Name"), "default"=0.0, "attrib name"="stop_time" ("attribute"), "ref in"=w311) -> ("error out"=w313:errorcluster, "data"=w307:dbl, "ref out"=w312:i32)  [unwired: 2 in, 1 out]
                n157 = xnode "H5Dread.xnode"("type name (default)"="frametype", "dataset name (this)"=w297, "error in (no error)"=w306, "default"=w300, "ref in"=w305) -> ("error out"=w299:errorcluster, "data"=w304:string[], "ref out"=w303:i32)  [unwired: 1 in, 1 out]
                n158 = case shown="No Error" w313 {
                  tunnel: w307 -> [w450 _]
                  frame No Error {
                    "stop_time" <- w450
                  }
                  frame Error {
                  }
                }
                n159 = xnode "H5Dread.xnode"("type name (default)"="name", "dataset name (this)"=w297, "error in (no error)"=w299, "default"=w300, "ref in"=w303) -> ("error out"=w298:errorcluster, "data"=w301:string[], "ref out"=w302:i32)  [unwired: 1 in, 1 out]
                n160 = call <vilib>:"H5Gclose.vi"("error in (no error)"=w298, "group in"=w302) -> ("error out"=w319:errorcluster)  [unwired: 3 in]
                n161 = property on="image_data" class="Arr (strict)"() -> ("Value"=w330:u16[][][])  [unwired: 2 in, 2 out]
                n162 = call <vilib>:"H5Lexists.vi"("error in (no error)"=w319, "path"=w318, "ref in"=w311) -> ("error out"=w317:errorcluster, "exists?"=w315:bool, "path out"=w316:string, "ref out"=w314:T21)  [unwired: 1 in]
                n163 = property on="raw_list" class="MCListbox (strict)"() -> ("ItemNames"=w336:string[][])  [unwired: 2 in, 2 out]
                n164 = call <userlib>:"Fix Sequence.vi"("sequences"=w301, "shots"=w304, "old sequence list"=w336, "image_data"=w330, "keep?"="hold_frames") -> ("sequencer"=w334:T22, "held data"=w333:u16[][][])
                n165 = case shown="True" w315 {
                  tunnel: [w415 w423] -> w337
                  tunnel: w316 -> [_ w427]
                  tunnel: [_ w434] -> w332
                  tunnel: w314 -> [_ w428]
                  tunnel: w317 -> [w415 w426]
                  tunnel: w334 -> [_ w430]
                  frame False {
                    # "Group doesn't exist yet, this is a new shot"
                  }
                  frame True {
                    n166 = call <vilib>:"H5Gopen.vi"("error in (no error)"=w426, "name"=w427, "ref in"=w428) -> ("error out"=w421:errorcluster, "group out"=w422:T21)  [unwired: 4 in]
                    n167 = xnode "H5Aread.xnode"("error in (no error)"=w421, "default"=u8[] [1, 1], "attrib name"="binning" ("attrib_name"), "ref in"=w422) -> ("error out"=w420:errorcluster, "data"=w418:u8[], "ref out"=w419:i32)  [unwired: 2 in, 1 out]
                    n168 = Array To Cluster(array=w418) -> (cluster=w429:cluster{"data[0]":u8, "data[1]":u8})
                    n169 = call <userlib>:"Read_Exposures.vi"("ref in"=w419, "sequencer"=w430, "error in"=w420) -> ("ref out"=w425:i32, "ROI"=w433:T6, "loaded images"=w434:u16[][][], "error out"=w424:errorcluster)  [unwired: 1 in, 1 out]
                    n170 = local read "roi_capture"() -> (w432:T6)
                    n171 = local write "binning"(w429) -> ()
                    n172 = call <userlib>:"Validate_Rect_Default.vi"("rect"=w433, "default"=w432) -> ("out"=w431:T6)
                    n173 = local write "roi_capture"(w431) -> ()
                    n174 = call <vilib>:"H5Gclose.vi"("error in (no error)"=w424, "group in"=w425) -> ("error out"=w423:errorcluster)  [unwired: 3 in]
                  }
                }
                n175 = Build Array (concatenate)(w333, w332) -> (w331:u16[][][])
              }
              frame Error {
                n176 = Greater Than 0?(x=w455) -> (x > 0?=w454:bool)
                n177 = case shown="True" w454 {
                  tunnel: w453 -> [w458 _]
                  tunnel: [w458 w461] -> w452
                  frame False {
                  }
                  frame True {
                    n178 = local read "camera name"() -> (w459:string)
                    n179 = Concatenate Strings("Specified HDF has no instructions for camera " ("error message (\"\")"), w459) -> (w460:string)
                    n180 = call <vilib>:"Error Cluster From Error Code.vi"("error message (\"\")"=w460, "error code (0)"=6013) -> ("error out"=w461:errorcluster)  [unwired: 7 in]
                  }
                }
                n181 = local write "current file"("") -> ()
                n182 = local read "sequencer"() -> (w456:T11)
                n183 = property on="image_data" class="Arr (strict)"() -> ("Value"=w451:u16[][][])  [unwired: 2 in, 2 out]
              }
            }
            "sequencer" <- w271
            n184 = call <vilib>:"H5Fclose.vi"("error in (no error)"=w253, "ref"=w252) -> ("error out"=w249:errorcluster)  [unwired: 3 in]
            n185 = local write "image_data"(w272) -> ()
            n186 = Lossy Enqueue Element(queue=w248, element=w249) -> ()  [unwired: 1 in, 4 out]
            n187 = case shown="Error" w249 {
              tunnel: [w291 w294] -> _
              tunnel: w250 -> [w291 w293]
              frame No Error {
              }
              frame Error {
                n188 = local write "current file"("") -> ()
                n189 = Flush Queue(queue=w293) -> (queue out=w294:refnum<queue>)  [unwired: 1 in, 2 out]
              }
            }
            n190 = for {
              tunnel: w271 -> [w287] mode=indexing
              tunnel: [w284] -> w270 mode=indexing
              shift-right: [w281] -> w269
              shift-left: string[][] [] -> [w280]
              n191 = Unbundle(w287) -> ("name"=w282:string, "shots"=w283:string[])  [unwired: 1 out]
              n192 = Equal?(x=w282, y="(held)") -> (x = y?=w285:bool)
              n193 = for {
                tunnel: w283 -> [w290] mode=indexing
                tunnel: w282 -> [w289]
                tunnel: [w288] -> w279 mode=indexing
                n194 = Build Array(w289, w290) -> (w288:string[])
              }
              n195 = Boolean To (0,1)(Boolean=w285) -> (0, 1=w284:i16)
              n196 = Build Array (concatenate)(w279, w280) -> (w281:string[][])
            }
            n197 = call <vilib>:"Clear Errors.vi"("error in (no error)"=w249) -> ("error out"=w262:errorcluster)  [unwired: 6 in]
            n198 = Merge Errors(w259, w262) -> (w261:errorcluster)
            n199 = call-dynamic "ZLockRelease.vi"("error in (no error)"=w261, "key"=w263, "ZLock in"=w264) -> ()  [unwired: 6 in, 3 out]
            n200 = Add Array Elements(numeric array=w270) -> (sum=→"keep":i16)
            n201 = property on="raw_list" class="MCListbox (strict)"("ItemNames"=w269) -> ()  [unwired: 2 in, 2 out]
          }
          frame "" {
            n202 = call <userlib>:"BasicLogger.vi"("text"="Empty \"read file\" command") -> ()  [unwired: 6 in, 2 out]
          }
        }
      }
      frame "Save File" {
        n203 = local read "working dir"() -> (w470:path)
        n204 = local read "current file"() -> (w469:string)
        n205 = Get Queue Status(queue=w467) -> ()  [unwired: 2 in, 8 out]
        n206 = case shown="Default" w469 {
          selector: w469 -> [w489 _]
          tunnel: w470 -> [w490 _]
          tunnel: [w478 w561] -> w465
          tunnel: w468 -> [w485 _]
          tunnel: [w483 _] -> _
          frame Default {
            n207 = Build Path(base path=w490, name or relative path=w489) -> (appended path=w481:path)
            n208 = Path To String(path=w481) -> (string=w488:string)
            n209 = local read "location"() -> (w492:string)
            n210 = call-dynamic "ZLockAcquire.vi"("key"=w488, "ZLock in"=w485) -> ("error out"=w480:errorcluster, "key out"=w486:string, "ZLock out"=w484:refnum<class "ZLock.lvclass">)  [unwired: 7 in]
            n211 = Concatenate Strings("Save file  " ("text"), w489) -> (w493:string)
            n212 = call <vilib>:"H5Fopen.vi"("error in (no error)"=w480, "mode (read-only)"=H5Fmode."read-write", "path"=w481) -> ("error out"=w472:errorcluster, "ref out"=w477:T21)  [unwired: 3 in]
            n213 = Concatenate Strings("images/" ("attribute"), w492) -> (w476:string)
            n214 = call <userlib>:"BasicLogger.vi"("text"=w493) -> ()  [unwired: 6 in, 2 out]
            n215 = call <vilib>:"H5Gopen.vi"("create? (F)"=TRUE, "error in (no error)"=w472, "name"=w476, "ref in"=w477) -> ("error out"=w475:errorcluster, "group out"=w474:T21)  [unwired: 3 in]
            n216 = case shown="No Error" w475 {
              selector: w475 -> [_ w558]
              tunnel: [w504 w558] -> w479
              tunnel: w474 -> [w503 _]
              frame No Error {
                n217 = property on="rois" class="Arr (strict)"() -> ("Value"=w502:T7)  [unwired: 2 in, 2 out]
                n218 = local read "effective_pixel"() -> (w508:dbl)
                n219 = local read "camera name"() -> (w512:string)
                n220 = for {
                  tunnel: w503 -> [w530]
                  tunnel: w502 -> [w522] mode=indexing
                  tunnel: [w528] -> w495
                  shift-right: [w527] -> w501
                  shift-left: _ -> [w526]
                  i -> [w525]
                  n221 = Unbundle(w522) -> ("rect"=w521:T6)  [unwired: 3 out]
                  n222 = Format Into String(format string="roi%d", w525) -> (resulting string=w523:string)  [unwired: 2 in, 1 out]
                  n223 = call <userlib>:"Validate_Rect.vi"("rect"=w521) -> ("valid"=w520:bool)
                  n224 = case shown="True" w520 {
                    tunnel: w530 -> [w532 w539]
                    tunnel: TRUE ("overwrite? (F)") -> [_ w535]
                    tunnel: [w532 w533] -> w528
                    tunnel: [w531 w534] -> w527
                    tunnel: w526 -> [w531 w538]
                    tunnel: w523 -> [_ w536]
                    tunnel: w521 -> [_ w537]
                    frame False {
                    }
                    frame True {
                      n225 = xnode "H5Awrite.xnode"("replace? (T)"=w535, "error in (no error)"=w538, "data"=w537, "attrib name"=w536, "ref in"=w539) -> ("error out"=w534:errorcluster, "ref out"=w533:i32)  [unwired: 2 in, 1 out]
                    }
                  }
                }
                n226 = local read "attribs"() -> (w510:variant[])
                n227 = call <userlib>:"Set Data Name__ogtk.vi"("Data Name"="effective_pixel_size", "Data"=w508) -> ("Renamed Data"=w506:variant)  [unwired: 8 in, 1 out]
                n228 = call <userlib>:"Set Data Name__ogtk.vi"("Data Name"="camera", "Data"=w512) -> ("Renamed Data"=w509:variant)  [unwired: 8 in, 1 out]
                n229 = Build Array (concatenate)(w506, w510, w509) -> (w497:variant[])
                n230 = for {
                  tunnel: w497 -> [w517] mode=indexing
                  tunnel: [w518] -> w498
                  shift-right: [w519] -> w496
                  shift-left: w495 -> [w513]
                  n231 = call <userlib>:"Get Data Name__ogtk.vi"("Data"=w517) -> ("Data Name"=w515:string, "Data dup"=w516:variant)  [unwired: 8 in, 1 out]
                  n232 = call <vilib>:"H5Awrite_var.vi"("replace? (T)"=FALSE ("overwrite?"), "data"=w516, "attrib name"=w515, "ref in"=w513) -> ("error out"=w518:errorcluster, "ref out"=w519:T21)  [unwired: 4 in, 1 out]
                }
                n233 = property on="sequencer" class="Arr (strict)"() -> ("Value"=w499:T11)  [unwired: 2 in, 2 out]
                n234 = property on="image_data" class="Arr (strict)"() -> ("Value"=w500:u16[][][])  [unwired: 2 in, 2 out]
                n235 = call <vilib>:"Clear Errors.vi"("error in (no error)"=w498) -> ()  [unwired: 6 in, 1 out]
                n236 = call <userlib>:"Write_raw_data.vi"("image_data"=w500, "sequencer"=w499, "ref in"=w496) -> ("error out"=w505:errorcluster)  [unwired: 3 in, 1 out]
                n237 = Merge Errors(w505, w501) -> (w504:errorcluster)
              }
              frame Error {
              }
            }
            n238 = call <vilib>:"H5Fclose.vi"("error in (no error)"=w479, "ref"=w477) -> ("error out"=w478:errorcluster)  [unwired: 3 in]
            n239 = call <vilib>:"Clear Errors.vi"("error in (no error)"=w478) -> ("error out"=w487:errorcluster)  [unwired: 6 in]
            n240 = Merge Errors(w480, w487) -> (w482:errorcluster)
            n241 = call-dynamic "ZLockRelease.vi"("error in (no error)"=w482, "key"=w486, "ZLock in"=w484) -> ("error out"=w483:errorcluster)  [unwired: 6 in, 2 out]
          }
          frame "" {
            n242 = call <vilib>:"Error Cluster From Error Code.vi"("error message (\"\")"="Cannot save file - no filename specified" ("error message (\"\")"), "error code (0)"=6015) -> ("error out"=w561:errorcluster)  [unwired: 7 in]
          }
        }
        n243 = Lossy Enqueue Element(queue=w466, element=w465) -> ()  [unwired: 1 in, 4 out]
      }
    }
  }
  n244 = while {
    tunnel: w6 -> [w563]
    tunnel: w37 -> [w564]
    stop <- FALSE stop-if-true
    n245 = event shown="[7] \"capture\": Value Change" {
      selector: _ -> [_ _ _ _ _ _ _ _ _ _ _ _ _ _]
      dyn-events: _ -> [_ _ _ _ _ _ _ _ _ _ _ _ _ _]
      timeout: 200 -> [_ _ _ _ _ _ _ _ _ _ _ _ _ _]
      tunnel: w564 -> [_ _ w586 w589 w632 _ _ w702 _ _ _ _ _ _]
      tunnel: w563 -> [w566 _ _ _ w631 _ _ w701 _ _ _ _ _ _]
      event Timeout {
        w568 = 4 items=["None", "Selection Tool", "Point Tool", "Line Tool", "Rectangle Tool", "Oval Tool", "Polygon Tool", "ClosedFreehandTool", "Annulus Tool", "Rotated Rectangle Tool", "Zoom Tool", "Pan Tool", "Polyline Tool", "Freehand Tool"] ("Tool")
        n246 = event-data() -> ()  [unwired: 1 in, 2 out]
        n247 = invoke on="img_OD" class="ImageControl" method="Get Last Event"("Which Events"=i32[] [2, 1]) -> ("Tool"=w569:i32)  [unwired: 7 in, 7 out]
        n248 = Equal?(x=w569, y=w568) -> (x = y?=w567:bool)
        n249 = case shown="False" w567 {
          tunnel: w566 -> [_ _]
          frame False {
          }
          frame True {
            n250 = local read "binning"() -> (w571:cluster{"x":u8, "y":u8})
            n251 = property on="img_OD" class="ImageControl"() -> ("ROI"=w577:T24)  [unwired: 2 in, 2 out]
            n252 = call <userlib>:"ROI_to_rects.vi"("binning"=w571, "ROI"=w577) -> ("rect"=w576:T6)  [unwired: 3 out]
            n253 = local read "roi_capture"() -> (w575:T6)
            n254 = local read "roi_capture"() -> (w573:T6)
            n255 = call <userlib>:"Apply_Rect_Offset.vi"("offset rect"=w575, "input"=w576) -> ("output"=w574:T6)  [unwired: 3 in]
            n256 = call <userlib>:"Clip_Rect.vi"("bounds"=w573, "rect"=w574) -> ("result"=w572:T6)  [unwired: 1 in]
            n257 = property on="roi_current" class="Clust (strict)"("Val(Sgnl)"=w572) -> ()  [unwired: 2 in, 2 out]
          }
        }
      }
      event Value Change {
        # "Something with interrupts to improve flicker"
        n258 = event-data() -> ()  [unwired: 1 in, 5 out]
        n259 = local read "roi_capture"() -> (w583:T6)
        n260 = local read "roi_current"() -> (w579:T6)
        n261 = Negate(x=w583) -> (-x=w582:T6)
        n262 = local read "binning"() -> (w578:cluster{"x":u8, "y":u8})
        n263 = call <userlib>:"Apply_Rect_Offset.vi"("offset rect"=w582, "input"=w579) -> ("output"=w581:T6)  [unwired: 3 in]
        n264 = call <userlib>:"Rect_to_ROI.vi"("rect"=w581, "binning"=w578) -> ("ROI"=w580:T25)
        n265 = property on="img_OD" class="ImageControl"("ROI"=w580) -> ()  [unwired: 2 in, 2 out]
      }
      event "stop": Value Change {
        n266 = event-data() -> ()  [unwired: 1 in, 5 out]
        n267 = Flush Queue(queue=w586) -> (queue out=w584:refnum<queue>)  [unwired: 1 in, 2 out]
        n268 = Enqueue Element(queue=w584, element=Imaging_State."Quit") -> ()  [unwired: 2 in, 3 out]
      }
      event "files": Value Change {
        n269 = event-data() -> ("OldVal"=w591:T1, "NewVal"=w590:T1)  [unwired: 1 in, 3 out]
        n270 = Cluster To Array(cluster=w591) -> (array=w593:bool[])
        n271 = Cluster To Array(cluster=w590) -> (array=w592:bool[])
        n272 = call <userlib>:"Detect_Boolean_Change.vi"("NewVal"=w592, "OldVal"=w593) -> ("ButtonId"=w588:i32)  [unwired: 2 out]
        n273 = Greater Or Equal To 0?(x=w588) -> (x >= 0?=w587:bool)
        n274 = case shown="True" w587 {
          tunnel: w589 -> [_ w594]
          tunnel: w588 -> [_ w595]
          frame False {
          }
          frame True {
            n275 = local read "current file"() -> (w596:string)
            n276 = case shown="0, 1" w595 {
              selector: w595 -> [_ _ _ w605]
              tunnel: w596 -> [_ _ _ w611]
              tunnel: w594 -> [w597 w599 _ w606]
              frame 2 {
                n277 = Enqueue Element(queue=w597, element=Imaging_State."Save File") -> ()  [unwired: 2 in, 3 out]
              }
              frame 3 {
                n278 = Enqueue Element(queue=w599, element=Imaging_State."Compute") -> ()  [unwired: 2 in, 3 out]
              }
              frame Default {
              }
              frame 0, 1 {
                n279 = local read "working dir"() -> (w610:path)
                n280 = call "File Dialog"("start path"=w610, "prompt"="Select H5 File", "default name"=w611, "pattern (all files)"="*.h5", "pattern label"="HDF files") -> ("selected path"=w604:path, "error out"=w602:errorcluster)  [unwired: 7 in, 2 out]
                n281 = call <vilib>:"H5Fis_hdf.vi"("error in (no error)"=w602, "path"=w604) -> ("error out"=w601:errorcluster, "valid?"=w603:bool)  [unwired: 1 in, 1 out]
                n282 = case shown="False" w603 {
                  tunnel: w604 -> [_ w624]
                  tunnel: w606 -> [_ w623]
                  tunnel: w605 -> [_ w613]
                  tunnel: w601 -> [_ _]
                  frame False {
                    n283 = One Button Dialog(message="Chosen file is not a valid HDF5") -> ()  [unwired: 1 in, 1 out]
                  }
                  frame True {
                    n284 = Flush Queue(queue=w623) -> (queue out=w619:refnum<queue>, remaining elements=w622:T9[])  [unwired: 1 in, 1 out]
                    n285 = Strip Path(path=w624) -> (stripped path=w621:path, name=w620:string)
                    n286 = property on="working dir" class="Path"("Value"=w621) -> (error out=w616:errorcluster)  [unwired: 2 in, 1 out]
                    n287 = Array Size(array=w622) -> (size(s)=w614:i32)
                    n288 = property on="current file" class="Str"(error in=w616, "Value"=w620) -> (error out=w615:errorcluster)  [unwired: 1 in, 1 out]
                    n289 = Enqueue Element(queue=w619, element=Imaging_State."Read File", error in (no error)=w615) -> (queue out=w617:refnum<queue>)  [unwired: 1 in, 2 out]
                    n290 = case shown="Default" w614 {
                      frame 0 {
                      }
                      frame Default {
                        n291 = call <userlib>:"BasicLogger.vi"("text"="File open forced queue clear") -> ()  [unwired: 6 in, 2 out]
                      }
                    }
                    n292 = case shown="Default" w613 {
                      tunnel: w617 -> [w627 w628]
                      frame Default {
                        n293 = Enqueue Element(queue=w627, element=Imaging_State."Redraw") -> ()  [unwired: 2 in, 3 out]
                      }
                      frame 1 {
                        n294 = Enqueue Element(queue=w628, element=Imaging_State."Acquire") -> ()  [unwired: 2 in, 3 out]
                      }
                    }
                  }
                }
              }
            }
          }
        }
      }
      event "capture.abort": Value Change {
        n295 = event-data() -> ("NewVal"=w630:bool)  [unwired: 1 in, 4 out]
        n296 = case shown="True" w630 {
          tunnel: w632 -> [_ w637]
          tunnel: w631 -> [_ w636]
          tunnel: [_ w633] -> _
          frame False {
          }
          frame True {
            n297 = Flush Queue(queue=w637) -> (error out=w634:errorcluster)  [unwired: 1 in, 2 out]
            n298 = call-dynamic "CameraAbort.vi"("error in (no error)"=w634, "CameraBase in"=w636) -> ("error out"=w633:errorcluster)  [unwired: 8 in, 1 out]
            n299 = call <userlib>:"BasicLogger.vi"("text"="Abort signalled") -> ()  [unwired: 6 in, 2 out]
          }
        }
      }
      event "tools_zoom": Value Change {
        n300 = event-data() -> ("OldVal"=w641:T2, "NewVal"=w640:T2)  [unwired: 1 in, 3 out]
        n301 = control-ref of="img_OD"() -> (w638:refnum<vi>)
        n302 = Cluster To Array(cluster=w641) -> (array=w642:bool[])
        n303 = Cluster To Array(cluster=w640) -> (array=w643:bool[])
        n304 = call <userlib>:"Detect_Boolean_Change.vi"("NewVal"=w643, "OldVal"=w642) -> ("ButtonId"=w644:i32)  [unwired: 2 out]
        n305 = Build Array(w638) -> (w639:refnum<vi>[])
        n306 = for {
          tunnel: w644 -> [w646]
          tunnel: [w645] -> _ mode=indexing
          tunnel: w639 -> [w645] mode=indexing
          n307 = case shown="1" w646 {
            tunnel: w645 -> [w647 w665 w677 w685 _]
            frame 0 {
              n308 = property on="Property Node" class="ImageControl" props=["ROI", "Image Area Size", "Image Area Height", "Image Area Width"](reference=w647) -> (reference out=w648:refnum<vi>, "ROI"=w654:T24, "Image Area Height"=w653:u32, "Image Area Width"=w652:u32)  [unwired: 1 in, 2 out]
              n309 = Unbundle(w654) -> ("Global Rectangle"=w651:i32[], "Contours"=w650:T26)
              n310 = Empty Array?(array=w650) -> (empty?=w649:bool)
              n311 = case shown="False" w649 {
                tunnel: w653 -> [w663 _]
                tunnel: w652 -> [w662 _]
                tunnel: w651 -> [w659 _]
                tunnel: w648 -> [w655 _]
                frame False {
                  n312 = formula code="Zx=W/(R[2]-R[0]);\nZy=H/(R[3]-R[1]);\nCx=(R[2]+R[0])/2;\nCy=(R[3]+R[1])/2;"("R"=w659, "H"=w663, "W"=w662) -> ("Zx"=w657:dbl, "Zy"=w658:dbl, "Cx"=w661:dbl, "Cy"=w660:dbl)
                  n313 = Max & Min(x=w657, y=w658) -> (min(x,y)=w656:dbl)  [unwired: 1 out]
                  n314 = property on="Property Node" class="ImageControl"(reference=w655, "X Zoom"=w656, "Y Zoom"=w656, "Image Center X Position"=w661, "Image Center Y Position"=w660) -> ()  [unwired: 1 in, 2 out]
                }
                frame True {
                }
              }
            }
            frame 1 {
              w672 = sgl 1.2 ("x")
              # "Zoom to ROI if possible"
              n315 = property on="Property Node" class="ImageControl"(reference=w665) -> (reference out=w666:refnum<vi>, "X Zoom"=w673:sgl, "Y Zoom"=w674:sgl, "ROI"=w671:T24, "Image Center Position"=w667:cluster{"X":u32, "Y":u32})  [unwired: 1 in, 1 out]
              n316 = local read "binning"() -> (w664:cluster{"x":u8, "y":u8})
              n317 = call <userlib>:"ROI_to_rects.vi"("binning"=w664, "ROI"=w671) -> ("center"=w669:cluster{"x":i16, "y":i16}, "valid"=w670:bool)  [unwired: 2 out]
              n318 = Select(t=w669, s=w670, f=w667) -> (s? t:f=w668:cluster{"X":u32, "Y":u32})
              n319 = Multiply(x=w673, y=w672) -> (x*y=w676:sgl)
              n320 = Multiply(x=w674, y=w672) -> (x*y=w675:sgl)
              n321 = property on="Property Node" class="ImageControl"(reference=w666, "X Zoom"=w676, "Y Zoom"=w675, "Image Center Position"=w668) -> ()  [unwired: 1 in, 2 out]
            }
            frame 2 {
              w679 = sgl 1.2 ("x")
              n322 = property on="Property Node" class="ImageControl"(reference=w677) -> (reference out=w678:refnum<vi>, "X Zoom"=w681:sgl, "Y Zoom"=w682:sgl, "Image Center Position"=w680:cluster{"X":u32, "Y":u32})  [unwired: 1 in, 1 out]
              n323 = Divide(x=w681, y=w679) -> (x/y=w684:sgl)
              n324 = Divide(x=w682, y=w679) -> (x/y=w683:sgl)
              n325 = property on="Property Node" class="ImageControl"(reference=w678, "X Zoom"=w684, "Y Zoom"=w683, "Image Center Position"=w680) -> ()  [unwired: 1 in, 2 out]
            }
            frame 3 {
              n326 = property on="Property Node" class="ImageControl"(reference=w685, "Zoom to Fit Mode"=TRUE) -> ()  [unwired: 1 in, 2 out]
            }
            frame Default {
            }
          }
        }
      }
      event "tools_view": Value Change {
        n327 = event-data() -> ("OldVal"=w689:cluster{"sel":bool, "in":bool, "out":bool}, "NewVal"=w688:cluster{"sel":bool, "in":bool, "out":bool})  [unwired: 1 in, 3 out]
        n328 = Cluster To Array(cluster=w689) -> (array=w696:bool[])
        n329 = Cluster To Array(cluster=w688) -> (array=w695:bool[])
        n330 = call <userlib>:"Detect_Boolean_Change.vi"("NewVal"=w695, "OldVal"=w696) -> ("FinalVal"=w693:bool[], "SingleEvent"=w691:bool, "ButtonId"=w694:i32)
        n331 = Array To Cluster(array=w693) -> (cluster=w690:T27)
        n332 = Select(t=w690, s=w691, f=w689) -> (s? t:f=w687:cluster{"sel":bool, "in":bool, "out":bool})
        n333 = case shown="0" w694 {
          tunnel: [w697 w698 w699 w700] -> w692
          frame Default {
            n334 = property on="img_OD" class="ImageControl"() -> ("Current ROI Tool"=w697:u32)  [unwired: 2 in, 2 out]
          }
          frame 0 {
            w698 = u32 8 items=["No Selection", "Point", "Line", "Rectangle", "Oval", "Polygon", "Freehand Region", "Annulus", "Zoom", "Pan", "Broken Line", "Freehand Line", "Rotated Rectangle"] ("Tool (Point)")
          }
          frame 1 {
            w699 = u32 3 items=["No Selection", "Point", "Line", "Rectangle", "Oval", "Polygon", "Freehand Region", "Annulus", "Zoom", "Pan", "Broken Line", "Freehand Line", "Rotated Rectangle"] ("Tool (Point)")
          }
          frame 2 {
            w700 = u32 9 items=["No Selection", "Point", "Line", "Rectangle", "Oval", "Polygon", "Freehand Region", "Annulus", "Zoom", "Pan", "Broken Line", "Freehand Line", "Rotated Rectangle"] ("Tool (Point)")
          }
        }
        n335 = local write "tools_view"(w687) -> ()
        n336 = property on="img_OD" class="ImageControl"("Current ROI Tool"=w692) -> ()  [unwired: 2 in, 2 out]
      }
      event "capture": Value Change {
        n337 = event-data() -> ("OldVal"=w703:T3, "NewVal"=w704:T3)  [unwired: 1 in, 3 out]
        n338 = Cluster To Array(cluster=w703) -> (array=w707:bool[])
        n339 = Cluster To Array(cluster=w704) -> (array=w706:bool[])
        n340 = call <userlib>:"Detect_Boolean_Change.vi"("NewVal"=w706, "OldVal"=w707) -> ("ButtonId"=w705:i32)  [unwired: 2 out]
        n341 = case shown="Default" w705 {
          selector: w705 -> [w716 _]
          tunnel: w702 -> [w712 _]
          tunnel: w701 -> [w710 _]
          frame 0, 1 {
            n342 = local read "roi_current"() -> (w718:T6)
            n343 = local read "roi_sensor"() -> (w715:T6)
            n344 = Equal To 0?(x=w716) -> (x = 0?=w717:bool)
            n345 = call <userlib>:"Validate_Rect_Default.vi"("rect"=w718, "default"=w715) -> ("out"=w714:T6)
            n346 = Select(t=w714, s=w717, f=w715) -> (s? t:f=w709:T6)
            n347 = call-dynamic "CameraCheckROI.vi"("ROI_in"=w709, "CameraBase in"=w710) -> ("ROI_out"=w708:T6)  [unwired: 7 in, 2 out]
            n348 = property on="roi_capture" class="Clust (strict)"("Val(Sgnl)"=w708) -> (error out=w711:errorcluster)  [unwired: 2 in, 1 out]
            n349 = Enqueue Element(queue=w712, element=Imaging_State."Software trigger", error in (no error)=w711) -> ()  [unwired: 1 in, 3 out]
          }
          frame Default {
          }
        }
      }
      event Value Change {
        # "try to avoid infinite loop"
        n350 = event-data() -> ("CtlRef"=w729:refnum<vi>, "OldVal"=w722:T8, "NewVal"=w721:T8)  [unwired: 1 in, 2 out]
        n351 = Unbundle By Name(w721) -> ("col_scheme"=w725:u16)
        n352 = Unbundle By Name(w722) -> ("col_scheme"=w724:u16)
        n353 = Unbundle By Name(w721) -> ("val_max"=w728:sgl)
        n354 = Unbundle By Name(w722) -> ("val_max"=w727:sgl)
        n355 = Not Equal?(x=w722, y=w721) -> (x != y?=w719:bool)
        n356 = Equal?(x=w725, y=w724) -> (x = y?=w723:bool)
        n357 = Not Equal?(x=w728, y=w727) -> (x != y?=w730:bool)
        n358 = And(x=w719, y=w723) -> (x .and. y?=w720:bool)
        n359 = case shown="True" w730 {
          tunnel: w729 -> [_ w735]
          tunnel: [_ w736] -> w726
          tunnel: w721 -> [_ w733]
          frame False {
          }
          frame True {
            n360 = Bundle By Name(cluster=w733, "automax"=FALSE) -> (w734:T8)
            n361 = property class="Clust (strict)"(reference=w735, "Value"=w734) -> (error out=w736:errorcluster)  [unwired: 1 in, 1 out]
          }
        }
        n362 = case shown="True" w720 {
          tunnel: w726 -> [_ w732]
          frame False {
          }
          frame True {
            n363 = local read "frame"() -> (w731:i32)
            n364 = property on="frame" class="DigNum (strict)"(error in=w732, "Val(Sgnl)"=w731) -> ()  [unwired: 1 in, 2 out]
          }
        }
      }
      event Value Change {
        n365 = event-data() -> ("CtlRef"=w738:refnum<vi>, "NewVal"=w742:u16)  [unwired: 1 in, 3 out]
        n366 = property class="Ring (strict)"(reference=w738) -> ("Owner"=w744:refnum<vi>)  [unwired: 1 in, 2 out]
        n367 = local read "frame"() -> (w745:i32)
        n368 = control-ref of="raw_ctrls"() -> (w743:refnum<vi>)
        n369 = Equal?(x=w744, y=w743) -> (x = y?=w741:bool)
        n370 = Greater Or Equal To 0?(x=w745) -> (x >= 0?=w740:bool)
        n371 = Not Exclusive Or(1:w740, 2:w741) -> (0:w739:bool)
        n372 = case shown="True" w739 {
          tunnel: w742 -> [_ w749]
          tunnel: w738 -> [_ w746]
          frame False {
          }
          frame True {
            n373 = case shown="0" w749 {
              tunnel: [w753 w761 w762 w763 w765] -> w748
              tunnel: [w752 _ _ _ w764] -> w747
              tunnel: w746 -> [w751 _ _ _ _]
              frame Default {
                w753 = u32 5 items=["Grayscale", "Binary", "Gradient", "Rainbow", "Temperature", "User Defined"] ("Palette:Palette Type")
                n374 = property on="Property Node" class="Ring (strict)"(reference=w751) -> ("RingText.Text"=w750:string)  [unwired: 1 in, 2 out]
                n375 = Concatenate Strings(w750, ".tsv" ("string")) -> (w754:string)
                n376 = Build Path(base path=path "Z:/Temp/rgb gradients", name or relative path=w754) -> (appended path=w757:path)
                n377 = call-poly <vilib>:"Read From Spreadsheet File.vi"("file path (dialog if empty)"=w757) -> ("all rows"=w758:dbl[][])  [unwired: 6 in, 4 out]
                n378 = for {
                  tunnel: w758 -> [w760] mode=indexing
                  tunnel: [w759] -> w752 mode=indexing
                  n379 = Array To Cluster(array=w760) -> (cluster=w759:T28)
                }
              }
              frame 0 {
                w761 = u32 0 items=["Grayscale", "Binary", "Gradient", "Rainbow", "Temperature", "User Defined"] ("Palette:Palette Type")
              }
              frame 1 {
                w762 = u32 3 items=["Grayscale", "Binary", "Gradient", "Rainbow", "Temperature", "User Defined"] ("Palette:Palette Type")
              }
              frame 2 {
                w763 = u32 4 items=["Grayscale", "Binary", "Gradient", "Rainbow", "Temperature", "User Defined"] ("Palette:Palette Type")
              }
              frame 3 {
                n380 = property on="img_OD" class="ImageControl"() -> ("Palette Type"=w765:u32, "User Palette"=w764:cluster{"Red":u8, "Green":u8, "Blue":u8}[])  [unwired: 2 in, 2 out]
              }
            }
            n381 = property on="img_OD" class="ImageControl"("Palette Type"=w748, "User Palette"=w747) -> ()  [unwired: 2 in, 2 out]
          }
        }
      }
      event "last error.status": Value Change; "last error.status", "recent_error": Mouse Up {
        n382 = event-data() -> ("Type"=w770:T23, "CtlRef"=w766:refnum<vi>)  [unwired: 1 in, 2 out]
        n383 = Equal?(x=lveventtype."Mouse Up" ("Type"), y=w770) -> (x = y?=w768:bool)
        n384 = case shown="False" w768 {
          tunnel: [w772 FALSE ("recent_error")] -> w767
          tunnel: w766 -> [w771 _]
          frame False {
            n385 = property on="Property Node" class="Bool (strict)"(reference=w771) -> ("Value"=w772:bool)  [unwired: 1 in, 2 out]
          }
          frame True {
          }
        }
        "recent_error" <- w767
      }
      event "raw_list": Value Change {
        n386 = event-data() -> ("CtlRef"=w781:refnum<vi>, "OldVal"=w779:i32, "NewVal"=w780:i32)  [unwired: 1 in, 2 out]
        n387 = Greater Or Equal To 0?(x=w779) -> (x >= 0?=w778:bool)
        n388 = Not Equal?(x=w779, y=w780) -> (x != y?=w783:bool)
        n389 = Greater Or Equal To 0?(x=w780) -> (x >= 0?=w777:bool)
        n390 = And(x=w783, y=w777) -> (x .and. y?=w782:bool)
        n391 = Exclusive Or(1:w778, 2:w777) -> (0:w776:bool)
        n392 = case shown="True" w782 {
          tunnel: w781 -> [_ w793]
          tunnel: w780 -> [_ w792]
          tunnel: w776 -> [_ w788]
          tunnel: [_ w787] -> w775
          tunnel: [w784 w786] -> w774
          frame False {
            n393 = local read "frame"() -> (w784:i32)
          }
          frame True {
            # "Set the other one to -1"
            n394 = control-ref of="raw_list"() -> (w785:refnum<vi>)
            n395 = Equal?(x=w785, y=w793) -> (x = y?=w789:bool)
            n396 = Negate(x=w792) -> (-x=w794:i32)
            n397 = Decrement(x=w794) -> (x-1=w791:i32)
            n398 = Select(t=w792, s=w789, f=w791) -> (s? t:f=w786:i32)
            n399 = case shown="True" w788 {
              frame False {
              }
              frame True {
                n400 = control-ref of="col_scheme"() -> (w795:refnum<vi>)
                n401 = property class="Ring (strict)"(reference=w795) -> (reference out=w798:refnum<vi>, error out=w797:errorcluster, "Value"=w796:u16)  [unwired: 1 in]
                n402 = property class="Ring (strict)"(reference=w798, error in=w797, "Val(Sgnl)"=w796) -> ()  [unwired: 2 out]
              }
            }
            n403 = property class="MCListbox (strict)"(reference=w785, "Value"=-1) -> (error out=w787:errorcluster)  [unwired: 1 in, 1 out]
          }
        }
        n404 = property on="frame" class="DigNum (strict)"(error in=w775, "Val(Sgnl)"=w774) -> ()  [unwired: 1 in, 2 out]
      }
      event "rois": Value Change {
        n405 = event-data() -> ("CtlRef"=w800:refnum<vi>, "NewVal"=w802:T7)  [unwired: 1 in, 3 out]
        n406 = for {
          tunnel: w802 -> [w837] mode=indexing
          tunnel: [w834] -> w801 mode=indexing
          w835 = FALSE ("get")
          n407 = Unbundle(w837) -> ("get"=w842:bool, "set"=w841:bool, "rect"=w838:T6)  [unwired: 1 out]
          n408 = Build Array(w842, w841) -> (w840:bool[])
          n409 = Boolean Array To Number(Boolean array=w840) -> (number=w839:u32)
          n410 = case shown="Default" w839 {
            tunnel: w838 -> [w843 _ w845]
            tunnel: [w843 w844 w845] -> w836
            frame Default {
            }
            frame 1 {
              # "set using roi_current"
              n411 = local read "roi_current"() -> (w844:T6)
            }
            frame 2 {
              n412 = property on="roi_current" class="Clust (strict)"("Val(Sgnl)"=w845) -> ()  [unwired: 2 in, 2 out]
            }
          }
          n413 = Bundle(cluster=w837, "get"=w835, "set"=w835, "rect"=w836) -> (w834:T29)  [unwired: 1 in]
        }
        n414 = property class="Arr (strict)"(reference=w800, "Value"=w801) -> (error out=w799:errorcluster)  [unwired: 1 in, 1 out]
        n415 = flat-sequence {
          tunnel: w799 -> [_]
          frame #0 {
            n416 = local read "img_OD"() -> (w807:T4)
            n417 = call "IMAQ Clear Overlay"("Groups"=string[] ["roi"], "Image"=w807) -> ("error out"=w811:errorcluster, "Image Out"=w809:T4)  [unwired: 8 in]
            n418 = call <vilib>:"Clear Errors.vi"("error in (no error)"=w811) -> ()  [unwired: 6 in, 1 out]
            n419 = local read "roi_capture"() -> (w812:T6)
            n420 = Build Array (concatenate)("rois") -> (w806:T7)
            n421 = Negate(x=w812) -> (-x=w813:T6)
            n422 = property on="x" class="DigNum (strict)"() -> ("Value"=w804:u8)  [unwired: 2 in, 2 out]
            n423 = property on="y" class="DigNum (strict)"() -> ("Value"=w803:u8)  [unwired: 2 in, 2 out]
            n424 = Bundle("Value"=w804, "Value"=w803, "Value"=w804, "Value"=w803) -> (w814:T30)  [unwired: 1 in]
            n425 = for {
              tunnel: w806 -> [w822] mode=indexing
              shift-right: [w819] -> w810
              shift-left: w809 -> [w823]
              tunnel: w813 -> [w816]
              tunnel: w814 -> [w815]
              n426 = Unbundle By Name(w822) -> ("color"=w820:u32, "rect"=w817:T6)
              n427 = Not Equal?(x=u32 16777216, y=w820) -> (x != y?=w818:bool)
              n428 = case shown="True" w818 {
                tunnel: w823 -> [w824 w833]
                tunnel: w820 -> [_ w831]
                tunnel: [w824 w830] -> w819
                tunnel: w817 -> [_ w829]
                tunnel: w816 -> [_ w828]
                tunnel: w815 -> [_ w826]
                frame False {
                }
                frame True {
                  n429 = call <userlib>:"Apply_Rect_Offset.vi"("offset rect"=w828, "input"=w829) -> ("output"=w827:T6)  [unwired: 3 in]
                  n430 = Quotient & Remainder(x=w827, y=w826) -> (floor(x/y)=w825:T6)  [unwired: 1 out]
                  n431 = call "IMAQ Overlay Rectangle"("Color"=w831, "Group"="roi", "Rectangle"=w825, "Image"=w833) -> ("Image Out"=w830:T4)  [unwired: 6 in, 1 out]
                }
              }
            }
            n432 = local write "img_OD"(w810) -> ()
          }
        }
      }
      event "frame": Value Change {
        # "RAW DATA"
        # "redraw ROIs"
        # "Manually rescale to an I16"
        # "We've changed type, so switch color schemes"
        # "Do we actually have the frame we're supposed to show?"
        n433 = event-data() -> ("NewVal"=w853:i32, "OldVal"=w852:i32)  [unwired: 1 in]
        n434 = property on="image_data" class="Arr (strict)"() -> ("Value"=w856:u16[][][])  [unwired: 2 in, 2 out]
        n435 = Less Than 0?(x=w852) -> (x < 0?=w854:bool)
        n436 = Equal?(x=w853, y=w852) -> (x = y?=w850:bool)
        n437 = Array Size(array=w856) -> (size(s)=w849:i32[])
        n438 = Index Array(array=w849) -> (element=w848:i32)  [unwired: 1 in]
        n439 = Less?(x=w853, y=w848) -> (x < y?=w847:bool)
        n440 = Select(t=w853, s=w847, f=0) -> (s? t:f=w877:i32)
        n441 = Less Than 0?(x=w877) -> (x < 0?=w874:bool)
        n442 = local write "frame"(w877) -> ()
        n443 = Index Array(array=w856, index (dim 0)=w877) -> (element=w867:u16[][])  [unwired: 2 in]
        n444 = control-ref of="col_scheme"() -> (w876:refnum<vi>)
        n445 = control-ref of="raw_ctrls"() -> (w870:refnum<vi>)
        n446 = Exclusive Or(1:w854, 2:w874) -> (0:w875:bool)
        n447 = Or(x=w850, y=w875) -> (x .or. y?=w851:bool)
        n448 = case shown="True" w851 {
          tunnel: w876 -> [_ w881]
          frame False {
          }
          frame True {
            n449 = property class="Ring (strict)"(reference=w881) -> (reference out=w880:refnum<vi>, error out=w878:errorcluster, "Value"=w879:u16)  [unwired: 1 in]
            n450 = property class="Ring (strict)"(reference=w880, error in=w878, "Val(Sgnl)"=w879) -> ()  [unwired: 2 out]
          }
        }
        n451 = property class="Clust (strict)"(reference=w870) -> (reference out=w868:refnum<vi>, "Value"=w871:T31)  [unwired: 1 in, 1 out]
        n452 = Unbundle By Name(w871) -> ("automax"=w873:bool, "val_max"=w869:sgl, "val_min"=w872:sgl)
        n453 = Subtract(x=w867, y=w872) -> (x-y=w864:sgl[][])
        n454 = case shown="False" w873 {
          tunnel: [w882 w885] -> w860
          tunnel: w867 -> [_ w887]
          tunnel: w868 -> [_ w886]
          tunnel: w869 -> [w882 _]
          tunnel: w871 -> [_ w883]
          frame False {
          }
          frame True {
            # "Recompute maximum value"
            n455 = Array Max & Min(array=w887) -> (max value=w885:u16)  [unwired: 3 out]
            n456 = Bundle By Name(cluster=w883, "val_max"=w885) -> (w884:T31)
            n457 = property class="Clust (strict)"(reference=w886, "Value"=w884) -> ()  [unwired: 1 in, 2 out]
          }
        }
        n458 = Subtract(x=w860, y=w872) -> (x-y=w861:sgl)
        n459 = Divide(x=sgl 32767.0, y=w861) -> (x/y=w863:sgl)
        n460 = Multiply(x=w864, y=w863) -> (x*y=w865:sgl[][])
        n461 = local read "img_OD"() -> (w857:T4)
        n462 = To Word Integer(number=w865) -> (16bit integer=w855:i16[][])
        n463 = local read "rois"() -> (w859:T7)
        n464 = call "IMAQ ArrayToImage"("Image Pixels (I16)"=w855, "Image"=w857) -> ("error out"=w858:errorcluster, "Image Out"=w866:T4)  [unwired: 8 in]
        n465 = local write "img_OD"(w866) -> ()
        n466 = property on="rois" class="Arr (strict)"(error in=w858, "Val(Sgnl)"=w859) -> ()  [unwired: 1 in, 2 out]
      }
    }
  }
  n467 = while {
    tunnel: w36 -> [w896]
    tunnel: w6 -> [w890]
    tunnel: w37 -> [w889]
    tunnel: w9 -> [w888]
    stop <- FALSE stop-if-true
    # "Wait for TCP"
    # "Run forever"
    n468 = TCP Wait On Listener(11:w896) -> (0:w893:errorcluster, 1:w894:u16, 2:w895:string, 4:w891:refnum<k5>)  [unwired: 3 in, 1 out]
    n469 = Format Into String(format string=":%d", initial string=w895, w894) -> (resulting string=w897:string)  [unwired: 1 in, 1 out]
    n470 = case shown="No Error" w893 {
      selector: w893 -> [_ w1013]
      tunnel: w891 -> [w925 _]
      tunnel: w897 -> [w920 _]
      tunnel: w889 -> [w906 _]
      tunnel: w890 -> [w905 _]
      tunnel: w888 -> [w901 _]
      frame No Error {
        # "Receive data"
        n471 = TCP Read(connection ID=w925, bytes to read=1024, 7:T32."CRLF" ("mode (standard)"), 9:500 ("timeout ms (25000)")) -> (connection ID out=w917:refnum<k5>, data out=w922:string, error out=w919:errorcluster)  [unwired: 1 in]
        n472 = Dequeue Element(queue=w901, timeout in ms (-1)=0) -> (queue out=w899:refnum<queue>, element=w900:errorcluster)  [unwired: 1 in, 2 out]
        n473 = call <vilib>:"Trim Whitespace.vi"("string"=w922) -> ("trimmed string"=w921:string)  [unwired: 1 in]
        n474 = case shown="Default" w921 {
          selector: w921 -> [w969 _ _ _]
          tunnel: w920 -> [w968 _ _ _]
          tunnel: w919 -> [w959 _ _ _]
          tunnel: [_ "done\r\n" ("data in") "hello\r\n" ("data in") _] -> w909
          tunnel: w906 -> [w965 w1003 w1004 w1011]
          tunnel: w905 -> [w964 w1002 _ _]
          tunnel: [w963 w999 w1005 w1008] -> w907
          tunnel: [w962 w1000 w1004 w1007] -> w903
          tunnel: w900 -> [w961 w998 w1005 w1009]
          frame Default {
            # "check it's an HDF"
            n475 = Get Date/Time In Seconds() -> (seconds since 1Jan1904=w967:timestamp)
            n476 = String To Path(string=w969) -> (path=w960:path)
            n477 = Format Into String(format string="Received \"%s\" from %s at %T", w969, w968, w967) -> (resulting string=w966:string)  [unwired: 2 in, 1 out]
            n478 = call <vilib>:"H5Fis_hdf.vi"("error in (no error)"=w959, "path"=w960) -> ("valid?"=w958:bool)  [unwired: 1 in, 2 out]
            n479 = call <userlib>:"BasicLogger.vi"("text"=w966) -> ()  [unwired: 6 in, 2 out]
            n480 = case shown="True" w958 {
              tunnel: w960 -> [w974 w990]
              tunnel: w965 -> [w971 w992]
              tunnel: [w976 w982] -> w963
              tunnel: w964 -> [_ w991]
              tunnel: [w971 w980] -> w962
              tunnel: w961 -> [_ w978]
              frame False {
                n481 = Format Into String(format string="Received file \"%s\" not a valid HDF ", w974) -> (resulting string=w973:string)  [unwired: 2 in, 1 out]
                n482 = call <vilib>:"Error Cluster From Error Code.vi"("error message (\"\")"=w973, "error code (0)"=6042 ("t")) -> ("error out"=w976:errorcluster)  [unwired: 7 in]
              }
              frame True {
                n483 = call-dynamic "CameraAbort.vi"("CameraBase in"=w991) -> ("error out"=w981:errorcluster)  [unwired: 9 in, 1 out]
                n484 = call <vilib>:"Clear Errors.vi"("error in (no error)"=w981) -> ("error out"=w977:errorcluster)  [unwired: 6 in]
                n485 = Merge Errors(w977, w978) -> (w979:errorcluster)
                n486 = flat-sequence {
                  tunnel: w990 -> [w993]
                  tunnel: w989 -> [w994]
                  tunnel: [w994] -> w984
                  frame #0 {
                    n487 = Strip Path(path=w993) -> (stripped path=w996:path, name=w995:string)
                    n488 = local write "working dir"(w996) -> ()
                    n489 = local write "current file"(w995) -> ()
                  }
                }
                n490 = Flush Queue(queue=w992, error in (no error)=w979) -> (queue out=w988:refnum<queue>, error out=w989:errorcluster)  [unwired: 1 out]
                n491 = Enqueue Element(queue=w988, element=Imaging_State."Read File", error in (no error)=w984) -> (queue out=w986:refnum<queue>, error out=w983:errorcluster)  [unwired: 1 in, 1 out]
                n492 = Enqueue Element(queue=w986, element=Imaging_State."Acquire", error in (no error)=w983) -> (queue out=w980:refnum<queue>, error out=w982:errorcluster)  [unwired: 1 in, 1 out]
              }
            }
          }
          frame "abort" {
            # "BLACS signals abort"
            # "Kill the queue"
            # "Abort the camera"
            n493 = call-dynamic "CameraAbort.vi"("CameraBase in"=w1002) -> ("error out"=w997:errorcluster)  [unwired: 9 in, 1 out]
            n494 = Merge Errors(w998, w997) -> (w999:errorcluster)
            n495 = Flush Queue(queue=w1003) -> (queue out=w1000:refnum<queue>)  [unwired: 1 in, 2 out]
          }
          frame "hello" {
          }
          frame "done" {
            n496 = Enqueue Element(queue=w1011, element=Imaging_State."Save File", error in (no error)=w1009) -> (queue out=w1007:refnum<queue>, error out=w1008:errorcluster)  [unwired: 1 in, 1 out]
            n497 = call <userlib>:"BasicLogger.vi"("text"="Received \"done\" command") -> ()  [unwired: 6 in, 2 out]
          }
        }
        n498 = case shown="\"\"" w909 {
          selector: w909 -> [w938 _]
          tunnel: w917 -> [w939 w955]
          tunnel: [w939 w952] -> w913
          tunnel: [w938 "done\r\n"] -> w912
          tunnel: [w937 w941] -> w908
          tunnel: w907 -> [w937 w946]
          tunnel: w899 -> [_ w940]
          frame Default {
          }
          frame "" {
            # "Send acknowledge response"
            n499 = Dequeue Element(queue=w940, timeout in ms (-1)=20000, error in (no error)=w946) -> (element=w943:errorcluster, timed out?=w945:bool, error out=w944:errorcluster)  [unwired: 1 out]
            n500 = TCP Write(connection ID=w955, data in="ok\r\n", 9:500 ("timeout ms (25000)")) -> (connection ID out=w952:refnum<k5>, error out=w957:errorcluster)  [unwired: 1 in, 1 out]
            n501 = Merge Errors(w944, w943) -> (w942:errorcluster)
            n502 = call <vilib>:"Clear Errors.vi"("error in (no error)"=w957) -> ()  [unwired: 6 in, 1 out]
            n503 = Select(t=6040, s=w945, f=0 ("error code (0)")) -> (s? t:f=w949:i32)
            n504 = call <vilib>:"Error Cluster From Error Code.vi"("error in (no error)"=w942, "error message (\"\")"="Imaging system timed out" ("error message (\"\")"), "error code (0)"=w949) -> ("error out"=w941:errorcluster)  [unwired: 6 in]
          }
        }
        n505 = case shown="Error" w908 {
          selector: w908 -> [w932 _]
          tunnel: [w930 w936] -> w916
          tunnel: w912 -> [_ w936]
          tunnel: w903 -> [w928 _]
          tunnel: [w927 _] -> _
          tunnel: [_ TRUE] -> w904
          tunnel: w899 -> [w926 _]
          frame Error {
            w931 = T14 0 items=["no dialog", "OK message", "continue or stop message", "OK message + warnings", "continue/stop + warnings"] ("type of dialog (OK msg:1)")
            # "kill any commands in the queue"
            # "Check if any errors occurred\nIf they did, BLACS will want to know"
            n506 = Flush Queue(queue=w928) -> ()  [unwired: 1 in, 3 out]
            n507 = Flush Queue(queue=w926) -> ()  [unwired: 1 in, 3 out]
            n508 = call <vilib>:"Simple Error Handler.vi"("type of dialog (OK msg:1)"=w931, "error in (no error)"=w932) -> ("error out"=w929:errorcluster, "message"=w933:string)  [unwired: 3 in, 3 out]
            n509 = Concatenate Strings("ERROR: " ("string"), w933) -> (w930:string)
            n510 = call <userlib>:"BasicErrorLogger.vi"("error in"=w929) -> ("error out"=w927:errorcluster)  [unwired: 1 in, 1 out]
          }
          frame No Error {
          }
        }
        n511 = local write "remote"(w904) -> ()
        n512 = TCP Write(connection ID=w913, data in=w916, 9:500 ("timeout ms (25000)")) -> (connection ID out=w911:refnum<k5>, error out=w914:errorcluster)  [unwired: 1 in, 1 out]
        n513 = TCP Close Connection(connection ID=w911, error in (no error)=w914) -> (error out=w918:errorcluster)  [unwired: 1 in, 1 out]
        n514 = call <vilib>:"Clear Errors.vi"("error in (no error)"=w918) -> ()  [unwired: 6 in, 1 out]
      }
      frame Error {
        n515 = call <userlib>:"BasicErrorLogger.vi"("error in"=w1013) -> ()  [unwired: 1 in, 2 out]
      }
    }
  }
  n516 = Stop(stop? (T)=w39) -> ()
  "acquiring" <- w27
